vi "RT.vi"() -> ()   [LabVIEW 2015]
uses:
  _RT Global.vi
  Type/RT Loop Events.ctl
  Type/_RT Active Ch.ctl
  Type/_RT Mass Range.ctl
  Type/_RT Expt.ctl
  Type/_RT Parameter.ctl
  <vilib>/rvi/interface/nirviReadWriteControl/nirviReadWriteControl.xnode
  Type/_RW Status.ctl
  <vilib>/Utility/config.llb/NI_LVConfig.lvlib
  Type/_RT Res Type.ctl
  Type/_Run Mode.ctl
  <vilib>/Utility/config.llb/Write Key (Boolean).vi
  Type/_FPGA Indicator.ctl
  Type/_RT Serial Command.ctl
  <vilib>/NI_Real-Time Target Support.lvlib
  Type/_RT LED Num.ctl
  Type/_RT Instrument State.ctl
  Type/_LED States.ctl
  Type/_Pump Parameter.ctl
  Type/_LCD Line1 Msg.ctl
  Type/_LCD Line2 Msg.ctl
  Type/FPGA Typedef.ctl
  Type/_RT Command.ctl
  Type/TCP Packet Info.ctl
  Type/_RT Data.ctl
  FPGA Bitfiles/FPGA9607.lvbitx
  <vilib>/Utility/config.llb/Write Key (String).vi
  NiFpgaLv.dll
  <vilib>/Utility/error.llb/Error Cluster From Error Code.vi
  <vilib>/rvi/errors/niLvFpgaAdjustHostInterfaceError.vi
panel:
  in  "FW Version":string="1.7.0.170921.R"
  out "Speed":i32
  out "error":errorcluster
  out "LC Input Detected 3":bool
  out "LC Input Detected 2":bool
  in  "# Connections":u8
  out "RunMode":i32
  out "Running":bool
  out "Command":T1
  in  "Force Simulation (F)":bool
  out "Rt Loop Events":T2
  out "code":i32
  out "InstrState":T3=enum."Mass Spectrometer is Off"
  out "Fault":bool
  out "Ready":bool
  in  "RT Version":u32=2107170921
  out "FPGA Version":u32
  out "Time (s)":dbl
  out "Connected?":bool
  # "R&D"
  # "Run  Status"
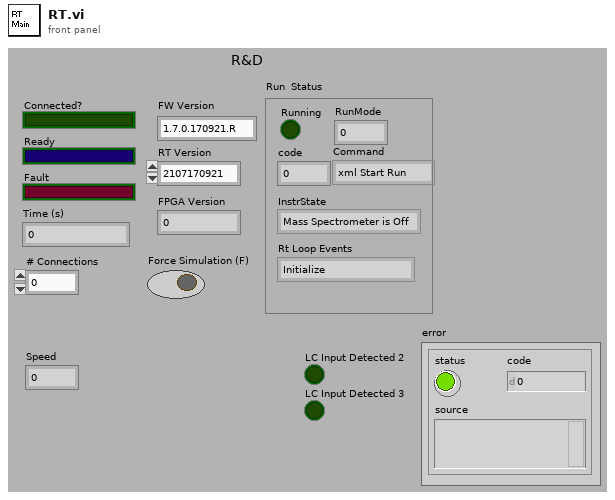
[diagram p1: front panel]
types:
  T1 = typedef "_RT Command.ctl" = enum16{"xml Start Run", "xml Start Actual Run", "xml Stop Run", "xml Runtime Update", "xml Get Status", "xml Get Table", "xml Set Table", "xml Get Configuration", "xml System Status", "xml Set LC Input Logic", "xml Get Data", "xml Get Info", "Start", "StartActualRun", "Stop", "Runtime Update", "Get Data", "Get Info", "Get Status", "Get Param", "Get Config", "Get Table", "Read ADC", "Set Oscillator", "Update Config", "Update Table", "Set All Pol", "Set Pol and DC", "Set Max Mass", "Toggle RP", "Toggle EL", "Set PIC", "Initialize Turbo", "Send Turbo Comm", "Close Turbo", "P1", "P2", "P3", "Send Serial", "Set LC Out", "Get LC In", "Read VAC", "Test Table", "Toggle Power", "Get Startup", "Set Startup", "Get ADC Table", "Set ADC Table", "Get Brief Status", "Get Detail Status", "Auxiliary Update", "Set CC Logics", "Set CC Input Logics", "Ignore Error", "invalid"}
  T2 = typedef "RT Loop Events.ctl" = enum16{"Initialize", "Wait for Connection", "Wait for Command", "Send Reply"}
  T3 = typedef "_RT Instrument State.ctl" = enum16{"Initializing", "Mass Spectrometer is Off", "Starting Up", "Turning Power Off", "Going to Standby", "Roughing Pump Ready", "Turning Turbo Off", "Turbo Startup", "Turbopump Ready", "Checking Vacuum", "Going to Ready", "Ready", "Running", "Source Standby", "Lost Communication", "Shutting Down", "Fault", "24V Standby", "Go to 24V Standby", "Turbopump Ready-Waiting"}
  T4 = typedef "_RT Parameter.ctl" = cluster{"RunMode":i32, "Initial Ch":T5[], "Sync":u8, "Expt":T6[], "EqTime(mS)":i32}
  T5 = typedef "_RT Active Ch.ctl" = cluster{"Start":i32, "Step":i32, "ChID":i32}
  T6 = typedef "_RT Expt.ctl" = cluster{"StartT(mS)":i32, "#Cycles":i32, "Scan Type":T7, "PauseT(uS)":i32, "Polarity":u8, "DelayT(mS)":i32, "Active Ch":T5[], "Mass Range":T8[]}
  T7 = typedef "_Run Mode.ctl" = enum16{"MRM (Q1/Q2)", "Q1 Scan", "Q1 SRM", "Q2 Scan", "Q2 SRM", "Product Scan", "Precursor Scan", "Neutral Loss", "Neutral Gain"}
  T8 = typedef "_RT Mass Range.ctl" = cluster{"Steps":i32, "Dwell(uS)":i32, "Resolution Type":T9, "Ramping Ch":T5[]}
  T9 = typedef "_RT Res Type.ctl" = u16
  T10 = cluster{"Rt Loop Events":T2, "Connection ID":refnum<k5>, "Parameter":T4, "Message Data":string, "Data Array":i32[], "Sequence Number":i32, "Command":T1, "error":errorcluster}
  T11 = typedef "FPGA Typedef.ctl" = refnum<k20>
  T12 = typedef "_RW Status.ctl" = enum8{"Done", "Do Read", "Do Write", "Set Latch1", "Set Latch2", "Set Latch3", "Set Latch4", "RP ON", "EL ON", "Serial Send", "Set LC Out", "Get LC In", "Read VAC", "Table Test", "Get Interlock", "Do Read2", "Do Write2"}
  T13 = typedef "_RT Serial Command.ctl" = cluster{"Port Type":u16, "baud rate (9600)":u32, "data bits (8)":u16, "stop bits (1)":u16, "parity (0:none)":u16, "DoRead":bool, "Command":string}
  T14 = typedef "_FPGA Indicator.ctl" = enum16{"Done", "Ready", "Count Available", "SendSerial", "LED State"}
  T15 = typedef "_Pump Parameter.ctl" = enum16{"Turn Pump Motor On", "Turn Pump Motor Off", "Read Pump Oil Deficiency", "Read Rotation Switch Point Attained", "Read Ele. Drive Over Temperature", "Read Pump Over Temperature", "Read Set Rotation Speed Attained", "Read Turbopump Accelerates", "Read Actual Rotation Speed in Hz", "Read Motor Current in A", "Read Operating Hours in h", "Read Motor Voltage in V", "Read Motor Power in W", "Set Rotation Speed Switchpoint in %", "Clear Error", "Read Error Code", "Read Bearing Temperature", "Read Hardware Version", "Read Firmware Version", "Read Operating Hours (Drive)", "Read Rotational Speed (rpm)", "Read Power Stage Temperature", "Read Electronics Temperature", "Read Upper Pump Temperature", "Read Motor Temperature", "Read Error Code History, 1", "Read Error Code History, 2", "Read Error Code History, 3", "Read Error Code History, 4", "Read Error Code History, 5", "Read Error Code History, 6", "Read Error Code History, 7", "Read Error Code History, 8", "Read Error Code History, 9", "Read Error Code History, 10"}
  T16 = typedef "TCP Packet Info.ctl" = cluster{"Packet Signature":string, "Sequence Number":i32, "Command":T1, "Data Message Size":u32, "Data Message Size":string, "Data Message":string, "Error Message Size":u32, "Error Message Size":string, "Error Message":string, "Checksum":u32, "Error Message":errorcluster, "Command ID":string}
  T17 = typedef "_RT Data.ctl" = cluster{"Info":string, "Data Array":i32[], "error out":errorcluster}
  T18 = typedef "_RT Startup Options.ctl" = cluster{"Door":bool, "Curtain":bool, "Pressure":bool, "Turbo":bool, "SysPoll":bool, "GasFlag":bool, "SourceExhaust":bool}
  T19 = typedef "_RT Instrument 2.ctl" = cluster{"Table":T20[], "Instrument":string[]}
  T20 = typedef "_RT Configuration 2.ctl" = cluster{"Name":string, "Ch#":u8, "Min":dbl, "Max":dbl, "Def+":dbl, "Def-":dbl, "Offset":dbl, "Slope":dbl, "Type":u8, "Description":string, "SettleT":dbl}
  T21 = typedef "NI_LVConfig.lvlib/Config Data RefNum.ctl" = refnum<k1>
  T22 = typedef "_RT LED Num.ctl" = enum8{"ReadKey", "ClearKeyBuffer", "ClearLCD", "BacklightOn"}
  T23 = typedef "_LED States.ctl" = enum8{"Idle", "Solid B", "Solid R", "Solid P", "Off B", "Off R", "Off P", "Off BRP", "Off RP", "Flash R&P", "Flash P"}
  T24 = typedef "_LCD Line2 Msg.ctl" = u16
  T25 = typedef "_LCD Line1 Msg.ctl" = u16
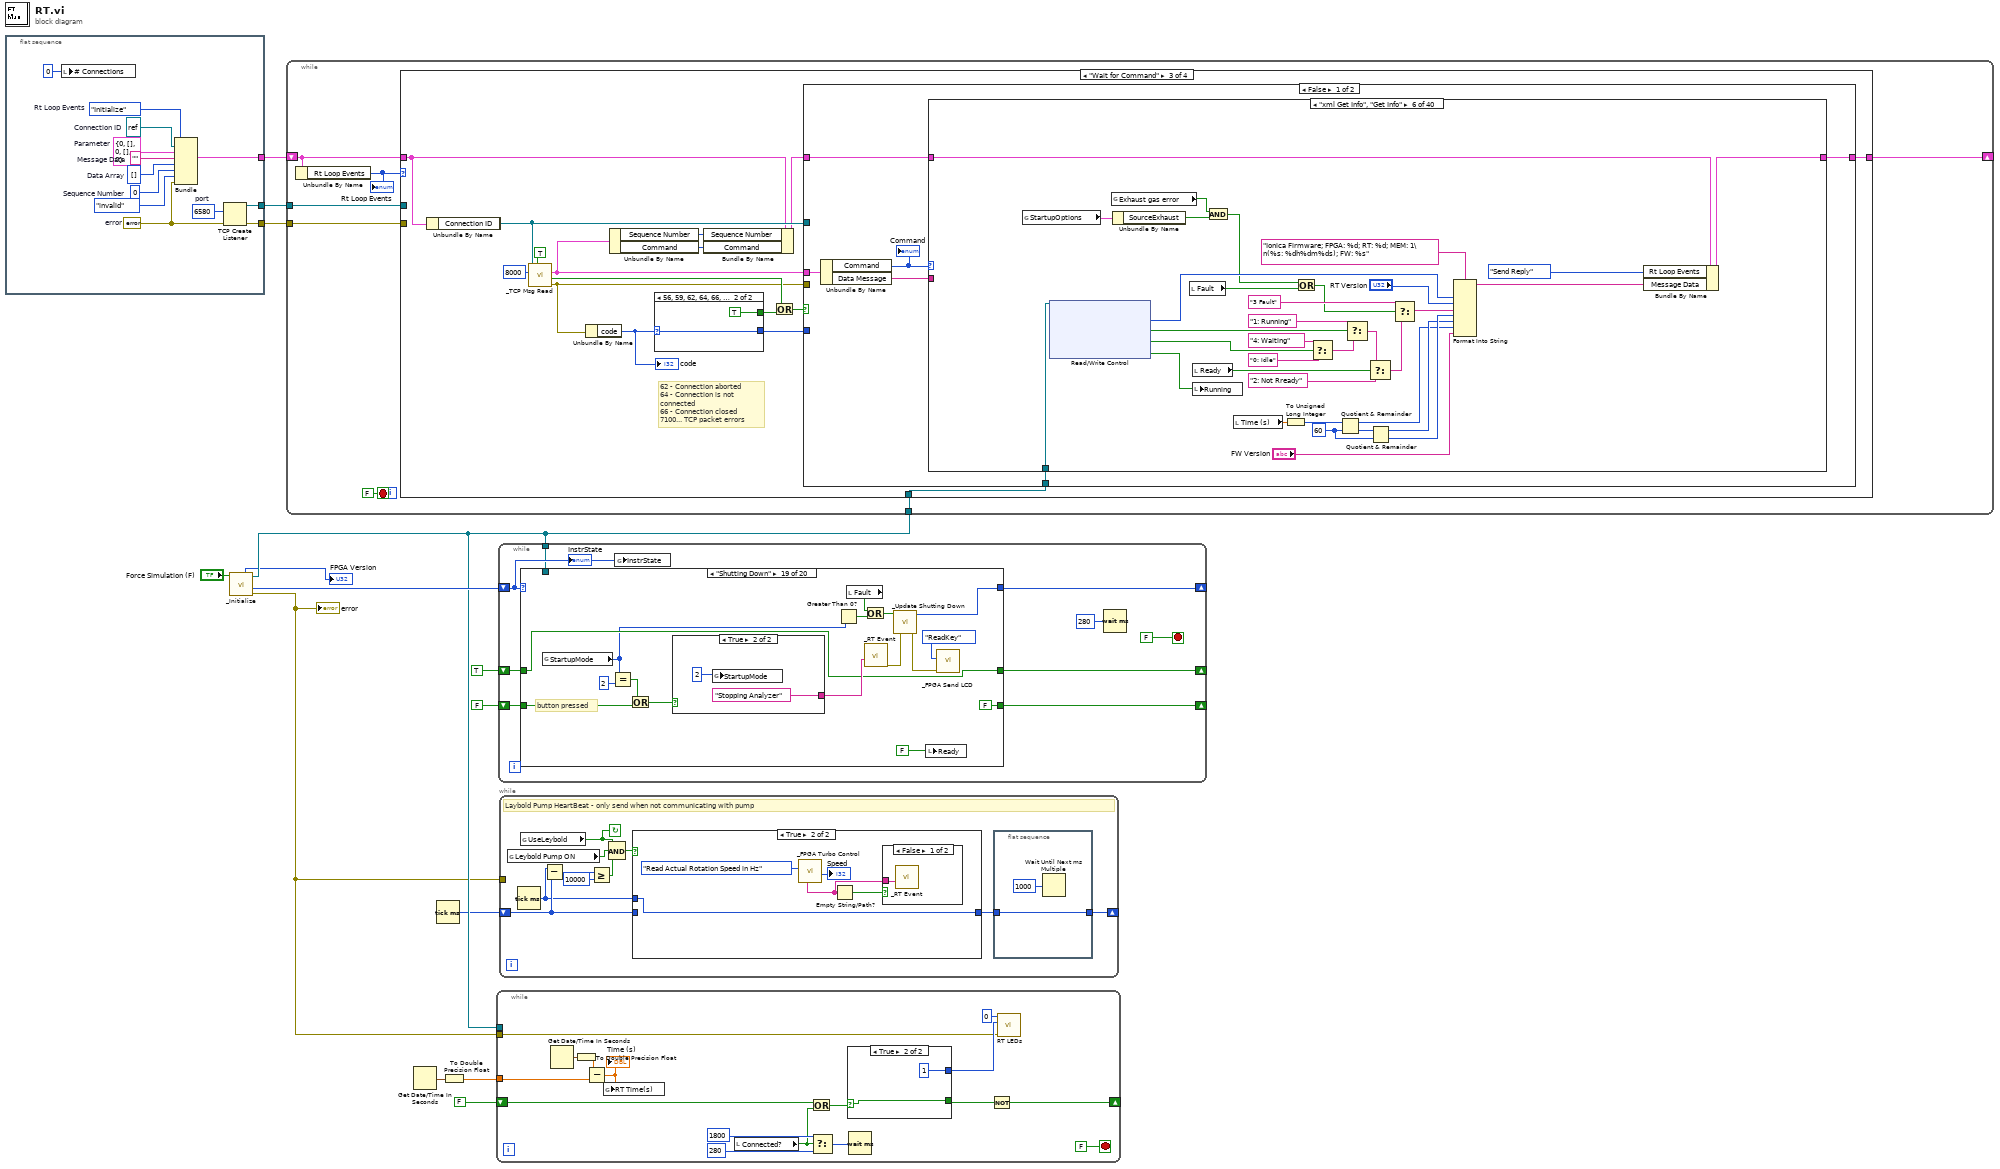
[diagram p0: block diagram]
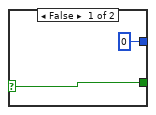
[diagram p4: hidden frame]
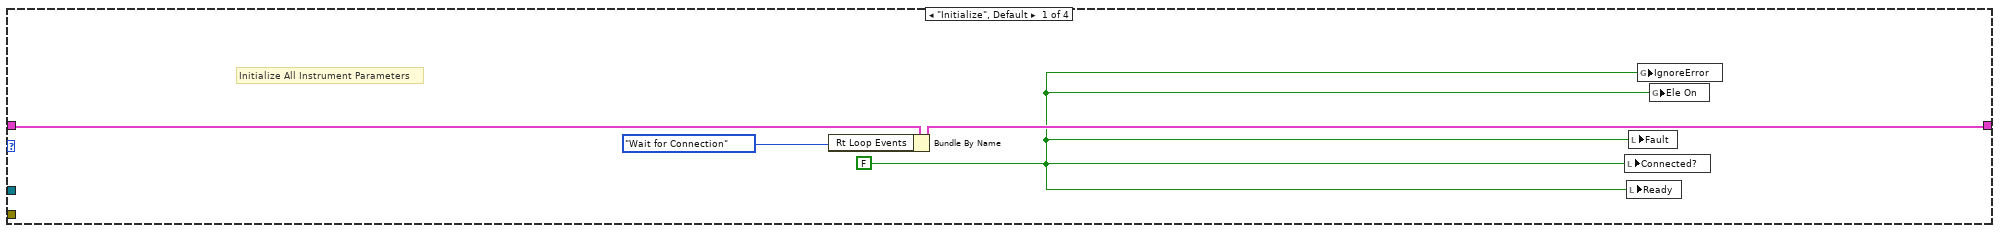
[diagram p5: hidden frame]
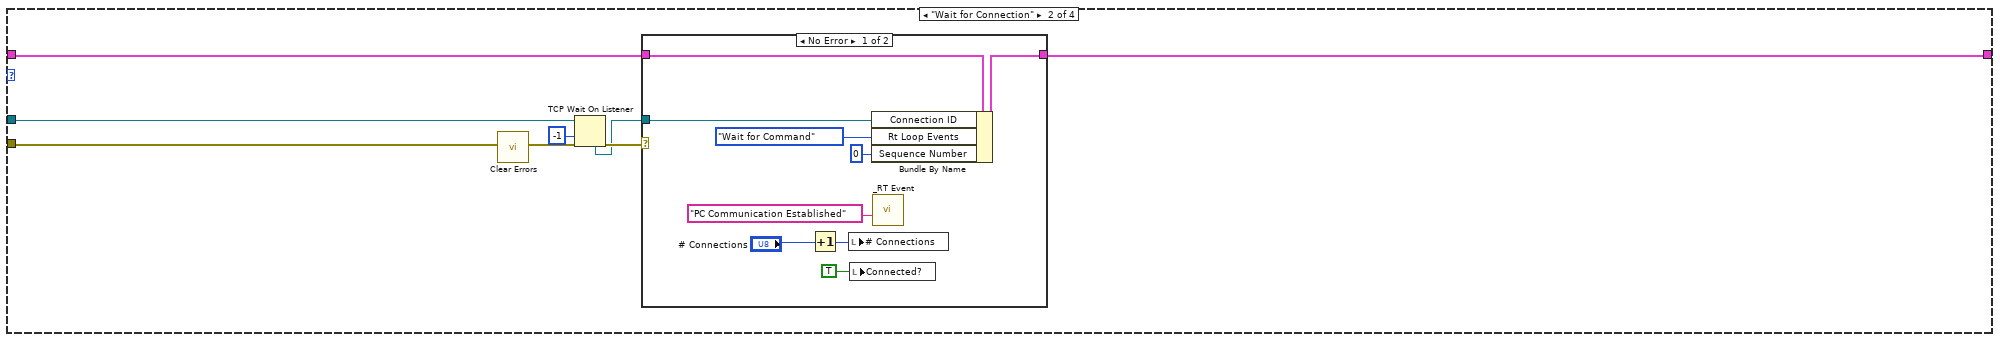
[diagram p6: hidden frame]
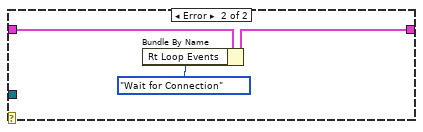
[diagram p7: hidden frame]
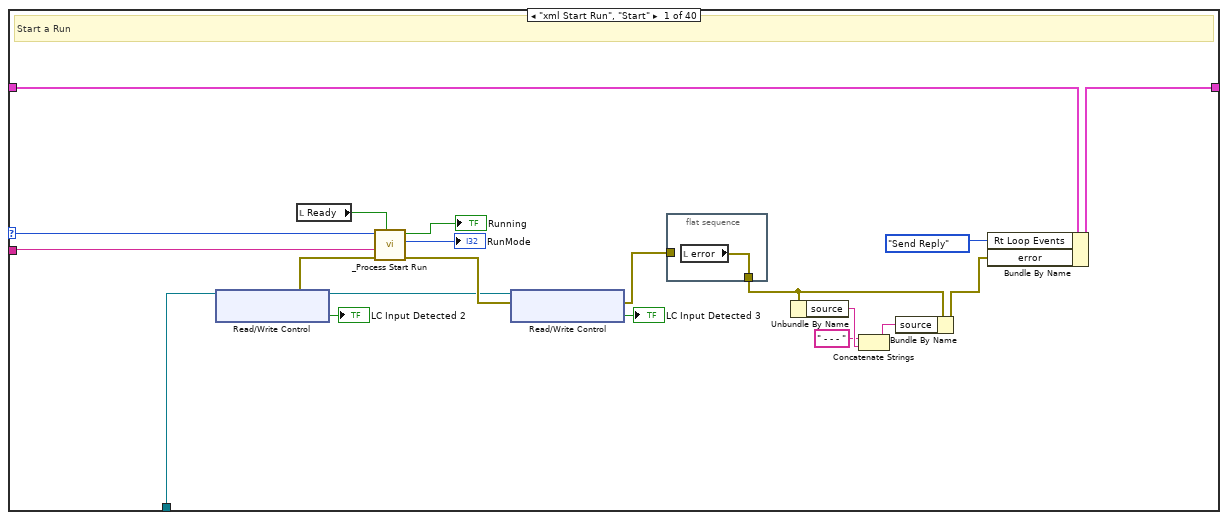
[diagram p8: hidden frame]
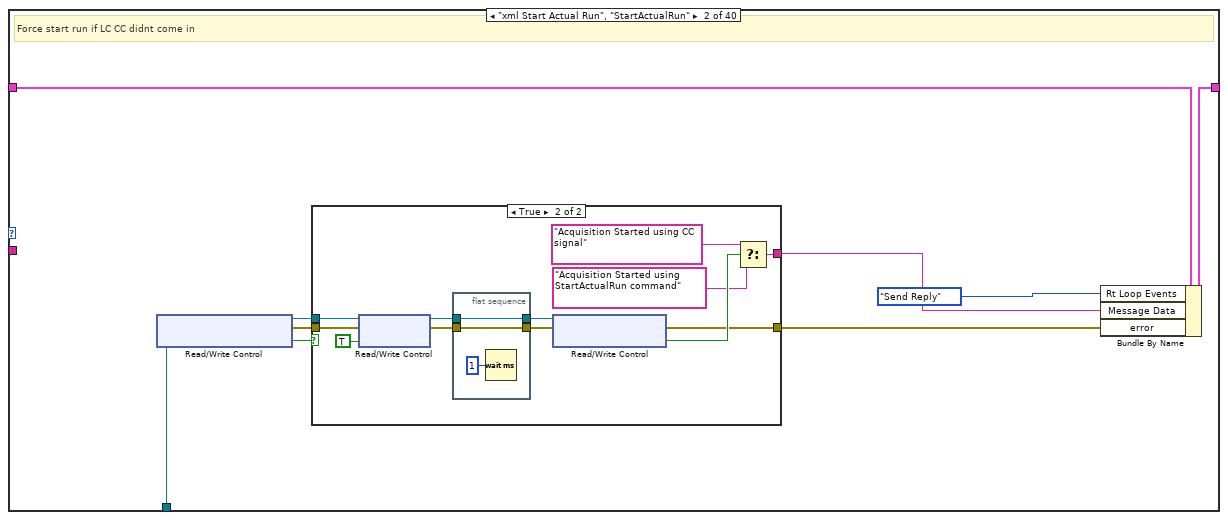
[diagram p9: hidden frame]
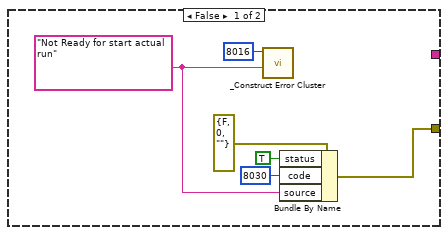
[diagram p10: hidden frame]
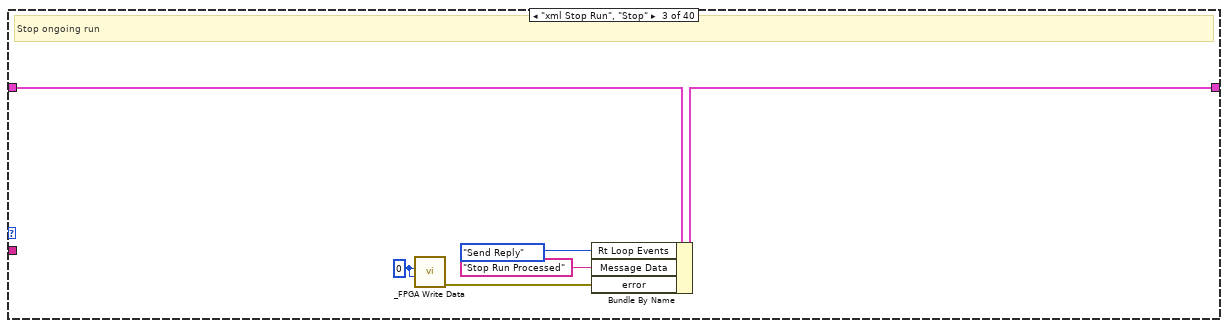
[diagram p11: hidden frame]
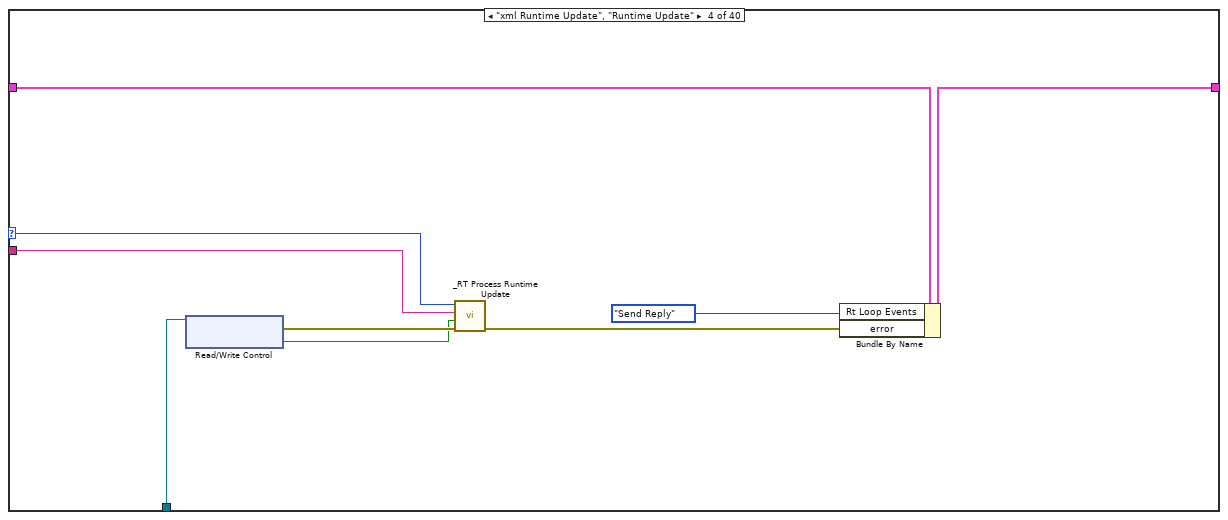
[diagram p12: hidden frame]
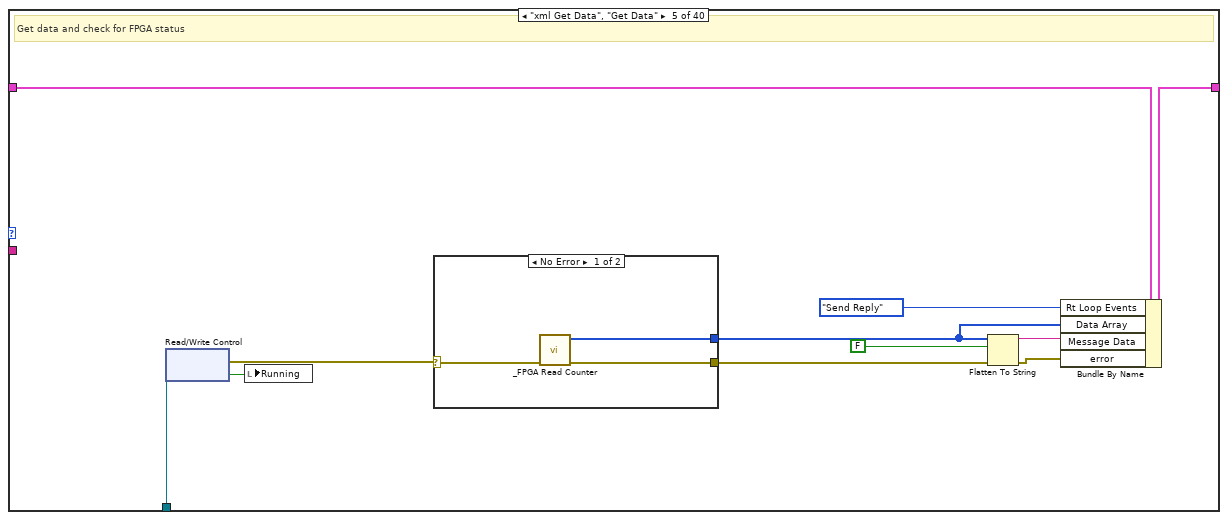
[diagram p13: hidden frame]
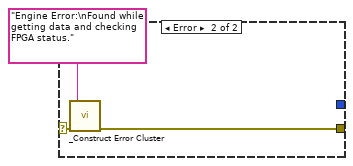
[diagram p14: hidden frame]
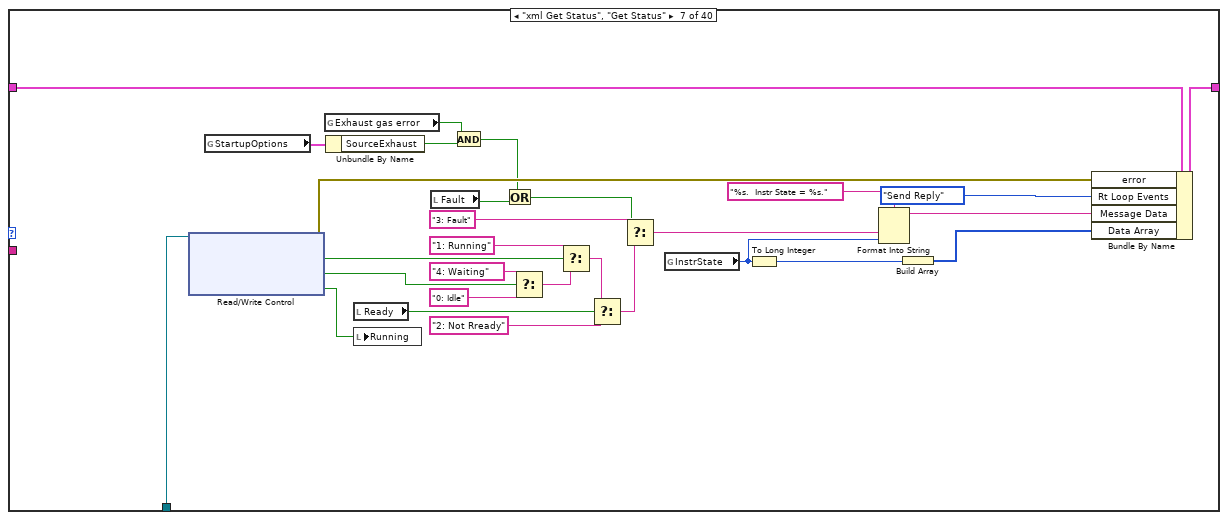
[diagram p15: hidden frame]
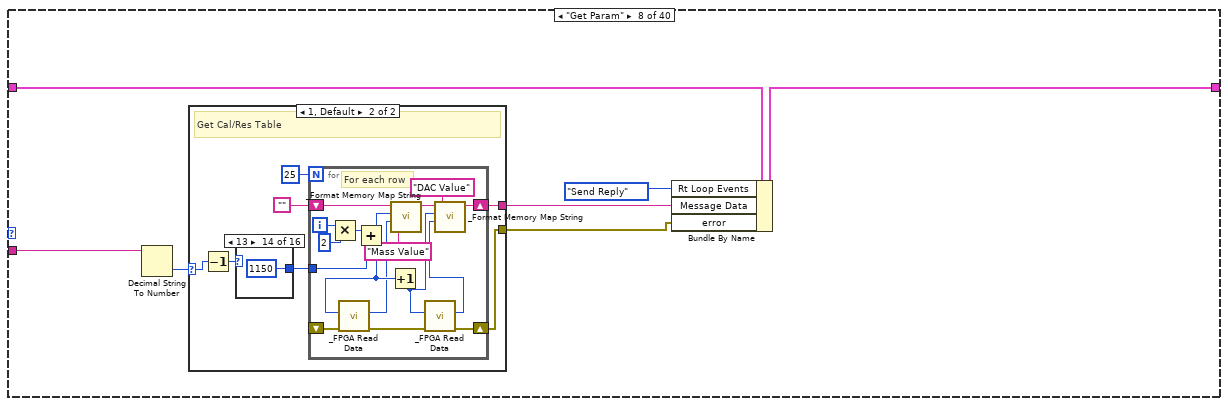
[diagram p16: hidden frame]
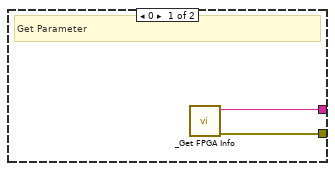
[diagram p17: hidden frame]
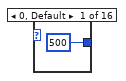
[diagram p18: hidden frame]
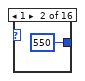
[diagram p19: hidden frame]
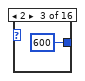
[diagram p20: hidden frame]
diagram:
  n1 = flat-sequence {
    tunnel: [w25] -> w14
    tunnel: [w21] -> w13
    tunnel: [w18] -> w5
    frame #0 {
      w19 = 0  # Sequence Number
      w20 = T4 {"RunMode"=0, "Initial Ch"=[], "Sync"=0, "Expt"=[], "EqTime(mS)"=0}  # Parameter
      w22 = u16 6580  # port
      w23 = i32[] []  # Data Array
      w24 = ""  # Message Data
      w15 = errorcluster {"status"=FALSE, "code"=0, "source"=""}  # error
      w26 = refnum<k5> refnum  # Connection ID
      w27 = RT_Loop_Events."Initialize"  # Rt Loop Events
      n2 = local write "# Connections"(u8 0 ("Disconnection#")) -> ()
      n3 = Bundle("Rt Loop Events"=w27, "Connection ID"=w26, "Parameter"=w20, "Message Data"=w24, "Data Array"=w23, "Sequence Number"=w19, "Command"=_RT_Command."invalid", "error"=w15) -> (w25:T10)  [unwired: 1 out]
      n4 = TCP Create Listener(8:w15, 10:w22) -> (0:w18:errorcluster, 3:w21:refnum<k5>)  [unwired: 4 out]
    }
  }
  n5 = call "_Initialize.vi"("Force Simulation (F)"="Force Simulation (F)") -> ("error"=w1:errorcluster, "InstrState"=w10:T3, "FPGA VI Reference Out"=w7:T11, "FPGA Version"=→"FPGA Version":u32)  [unwired: 7 in]
  "error" <- w1
  n6 = while {
    shift-right: [w28] -> _
    shift-left: w14 -> [w32]
    tunnel: w7 -> [w31]
    tunnel: w13 -> [w30]
    tunnel: w5 -> [w29]
    stop <- FALSE stop-if-true
    n7 = Unbundle By Name(w32) -> ("Rt Loop Events"=w33:T2)
    "Rt Loop Events" <- w33
    n8 = case shown="\"Wait for Command\"" w33 {
      tunnel: w32 -> [w37 w46 w59 w758]
      tunnel: [w36 w45 w73 w772] -> w28
      tunnel: w31 -> [_ _ w71 _]
      tunnel: w30 -> [_ w43 _ _]
      tunnel: w29 -> [_ w40 _ _]
      frame "Initialize", Default {
        w35 = FALSE ("Connected?")
        # "Initialize All Instrument Parameters"
        n9 = Bundle By Name(cluster=w37, "Rt Loop Events"=RT_Loop_Events."Wait for Connection") -> (w36:T10)
        n10 = local write "Connected?"(w35) -> ()
        n11 = local write "Ready"(w35) -> ()
        n12 = local write "Fault"(w35) -> ()
        n13 = global write "_RT Global.vi" "IgnoreError"(w35) -> ()
        n14 = global write "_RT Global.vi" "Ele On"(w35) -> ()
      }
      frame "Wait for Connection" {
        n15 = call <vilib>:"Clear Errors.vi"("error in (no error)"=w40) -> ("error out"=w39:errorcluster)  [unwired: 5 in, 1 out]
        n16 = TCP Wait On Listener(8:w39, 9:-1 ("timeout ms (wait forever: -1)"), 11:w43) -> (0:w44:errorcluster, 4:w42:refnum<k5>)  [unwired: 4 out]
        n17 = case shown="No Error" w44 {
          tunnel: w46 -> [w55 w58]
          tunnel: w42 -> [w53 _]
          tunnel: [w54 w56] -> w45
          frame No Error {
            n18 = Increment(x="# Connections") -> (x+1=w50:u8)
            n19 = local write "# Connections"(w50) -> ()
            n20 = local write "Connected?"(TRUE ("Connected?")) -> ()
            n21 = Bundle By Name(cluster=w55, "Connection ID"=w53, "Rt Loop Events"=RT_Loop_Events."Wait for Command", "Sequence Number"=0) -> (w54:T10)
            n22 = call "_RT Event.vi"("Event"="PC Communication Established") -> ()  [unwired: 2 in, 5 out]
          }
          frame Error {
            n23 = Bundle By Name(cluster=w58, "Rt Loop Events"=RT_Loop_Events."Wait for Connection") -> (w56:T10)
          }
        }
      }
      frame "Wait for Command" {
        # "62 - Connection aborted\n64 - Connection is not connected\n66 - Connection closed\n7100... TCP packet errors"
        n24 = Unbundle By Name(w59) -> ("Connection ID"=w69:refnum<k5>)
        n25 = call "_TCP Msg Read.vi"("RT"=TRUE, "timeout ms (10000)"=8000 ("millisecond multiple"), "connection ID"=w69) -> ("error out"=w60:errorcluster, "Read Timeout"=w66:bool, "Packet Info"=w62:T16)  [unwired: 1 in, 5 out]
        n26 = Unbundle By Name(w60) -> ("code"=w74:i32)
        "code" <- w74
        n27 = Unbundle By Name(w62) -> ("Sequence Number"=w64:i32, "Command"=w63:T1)
        n28 = case shown="56, 59, 62, 64, 66, 7100.., Default" w74 {
          selector: w74 -> [w753 w754]
          tunnel: [_ TRUE ("abort (F)")] -> w68
          tunnel: [w753 w754] -> w61
          frame 0 {
          }
          frame 56, 59, 62, 64, 66, 7100.., Default {
          }
        }
        n29 = Bundle By Name(cluster=w59, "Sequence Number"=w64, "Command"=w63) -> (w65:T10)
        n30 = Or(x=w66, y=w68) -> (x .or. y?=w70:bool)
        n31 = case shown="False" w70 {
          tunnel: w65 -> [w80 w733]
          tunnel: [w79 w732] -> w73
          tunnel: w62 -> [w77 _]
          tunnel: w71 -> [w78 _]
          tunnel: w69 -> [_ w731]
          tunnel: w61 -> [_ w730]
          tunnel: w60 -> [_ w729]
          frame False {
            n32 = Unbundle By Name(w77) -> ("Command"=w76:T1, "Data Message"=w75:string)
            "Command" <- w76
            n33 = case shown="\"xml Get Info\", \"Get Info\"" w76 {
              selector: w76 -> [w97 _ _ w140 _ _ _ _ w276 _ _ _ w337 w382 _ _ _ _ _ _ _ _ _ _ _ _ _ _ _ _ _ _ _ _ _ _ w694 _ _ w722]
              tunnel: w75 -> [w96 _ _ w141 _ _ _ w231 _ _ w300 w327 w340 w381 w404 w425 w429 w440 w455 w471 w479 w487 w499 w509 _ _ w546 w574 _ w587 _ w615 w622 _ w678 w689 w699 w712 w721 _]
              tunnel: w80 -> [w99 w109 w137 w145 w157 w198 w227 w234 w282 w294 w306 w324 w343 w386 w401 w422 w433 w442 w453 w468 w476 w484 w497 w513 w522 w529 w556 w577 w583 w597 w603 w612 w639 w672 w683 w692 w701 w715 w718 w725]
              tunnel: [w98 w108 w136 w144 w156 w197 w226 w233 w281 w293 w305 w323 w342 w384 w400 w421 w432 w441 w452 w467 w475 w483 w496 w512 w521 w528 w555 w576 w582 w596 w602 w611 w638 w671 w682 w691 w700 w714 w717 w724] -> w79
              tunnel: w78 -> [w92 w107 _ w143 w153 w195 w224 _ _ _ w304 _ _ _ _ _ _ _ w451 _ _ _ w495 _ _ _ w531 _ _ _ _ _ _ w656 _ _ _ _ _ _]
              frame "xml Start Run", "Start" {
                # "Start a Run"
                n34 = xnode "Read/Write Control"("FPGA VI Reference In"=w92) -> ("FPGA VI Reference Out"=w89:T11, "error out"=w91:errorcluster, "LC Input Detected"=→"LC Input Detected 2":bool)  [unwired: 1 in]
                n35 = local read "Ready"() -> (w95:bool)
                n36 = call "_Process Start Run.vi"("Ready"=w95, "Error In"=w91, "binary string"=w96, "Command"=w97) -> ("Error Out"=w90:errorcluster, "RunMode"=→"RunMode":i32, "Running"=→"Running":bool)  [unwired: 5 in]
                n37 = xnode "Read/Write Control"("FPGA VI Reference In"=w89, "error in"=w90) -> ("error out"=w85:errorcluster, "LC Input Detected"=→"LC Input Detected 3":bool)  [unwired: 1 out]
                n38 = flat-sequence {
                  tunnel: [w101] -> w84
                  tunnel: w85 -> [_]
                  frame #0 {
                    n39 = local read "error"() -> (w101:errorcluster)
                  }
                }
                n40 = Unbundle By Name(w84) -> ("source"=w83:string)
                n41 = Concatenate Strings(" - - - " ("string"), w83) -> (w82:string)
                n42 = Bundle By Name(cluster=w84, "source"=w82) -> (w86:errorcluster)
                n43 = Bundle By Name(cluster=w99, "Rt Loop Events"=RT_Loop_Events."Send Reply", "error"=w86) -> (w98:T10)
              }
              frame "xml Start Actual Run", "StartActualRun" {
                # "Force start run if LC CC didnt come in"
                n44 = xnode "Read/Write Control"("FPGA VI Reference In"=w107) -> ("FPGA VI Reference Out"=w104:T11, "error out"=w105:errorcluster, "Ready to Acquire Data"=w106:bool)  [unwired: 1 in]
                n45 = case shown="True" w106 {
                  tunnel: w105 -> [_ w126]
                  tunnel: w104 -> [_ w128]
                  tunnel: [w111 w118] -> w103
                  tunnel: [_ w117] -> w102
                  frame False {
                    w112 = "Not Ready for start actual run"
                    n46 = call "_Construct Error Cluster.vi"("reason"=w112, "errorCode"=8016) -> ()  [unwired: 2 in, 4 out]
                    n47 = Bundle By Name(cluster=errorcluster {"status"=FALSE, "code"=0, "source"=""} ("error constant"), "status"=TRUE, "code"=8030, "source"=w112) -> (w111:errorcluster)
                  }
                  frame True {
                    n48 = xnode "Read/Write Control"("FPGA VI Reference In"=w128, "error in"=w126, "ForceStart"=TRUE ("Start")) -> ("FPGA VI Reference Out"=w119:T11, "error out"=w121:errorcluster)
                    n49 = flat-sequence {
                      tunnel: [w131] -> w122
                      tunnel: w121 -> [w131]
                      tunnel: [w130] -> w120
                      tunnel: w119 -> [w130]
                      frame #0 {
                        n50 = Wait (ms)(milliseconds to wait=u32 1) -> ()  [unwired: 1 out]
                      }
                    }
                    n51 = xnode "Read/Write Control"("FPGA VI Reference In"=w120, "error in"=w122) -> ("error out"=w118:errorcluster, "LC Input Detected"=w125:bool)  [unwired: 1 out]
                    n52 = Select(t="Acquisition Started using CC signal" ("source"), s=w125, f="Acquisition Started using StartActualRun command" ("source")) -> (s? t:f=w117:string)
                  }
                }
                n53 = Bundle By Name(cluster=w109, "Rt Loop Events"=RT_Loop_Events."Send Reply", "Message Data"=w102, "error"=w103) -> (w108:T10)
              }
              frame "xml Stop Run", "Stop" {
                w134 = u16 0 ("Address")
                # "Stop ongoing run"
                n54 = call "_FPGA Write Data.vi"("Data"=w134, "Address"=w134) -> ("error out"=w133:errorcluster)  [unwired: 4 in, 2 out]
                n55 = Bundle By Name(cluster=w137, "Rt Loop Events"=RT_Loop_Events."Send Reply", "Message Data"="Stop Run Processed" ("string"), "error"=w133) -> (w136:T10)
              }
              frame "xml Runtime Update", "Runtime Update" {
                n56 = xnode "Read/Write Control"("FPGA VI Reference In"=w143) -> ("error out"=w142:errorcluster, "Acquiring Data"=w138:bool)  [unwired: 1 in, 1 out]
                n57 = call "_RT Process Runtime Update.vi"("Error In"=w142, "Acquiring Data"=w138, "binary string"=w141, "Command"=w140) -> ("Error Out"=w139:errorcluster)  [unwired: 7 in]
                n58 = Bundle By Name(cluster=w145, "Rt Loop Events"=RT_Loop_Events."Send Reply", "error"=w139) -> (w144:T10)
              }
              frame "xml Get Data", "Get Data" {
                # "Get data and check for FPGA status"
                n59 = xnode "Read/Write Control"("FPGA VI Reference In"=w153) -> ("error out"=w154:errorcluster, "Running"=w155:bool)  [unwired: 1 in, 1 out]
                n60 = local write "Running"(w155) -> ()
                n61 = case shown="No Error" w154 {
                  selector: w154 -> [w160 w163]
                  tunnel: [w158 _] -> w147
                  tunnel: [w159 w161] -> w150
                  frame No Error {
                    n62 = call "_FPGA Read Counter.vi"("error in (no error)"=w160) -> ("error out"=w159:errorcluster, "Data"=w158:u32[])  [unwired: 8 in, 1 out]
                  }
                  frame Error {
                    n63 = call "_Construct Error Cluster.vi"("error in"=w163, "reason"="Engine Error:\nFound while getting data and checking FPGA status.") -> ("error out"=w161:errorcluster)  [unwired: 2 in, 3 out]
                  }
                }
                n64 = Flatten To String(anything=w147, prepend array or string size? (T)=FALSE, error in (no error)=w150) -> (data string=w152:string, error out=w149:errorcluster)  [unwired: 1 in, 1 out]
                n65 = Bundle By Name(cluster=w157, "Rt Loop Events"=RT_Loop_Events."Send Reply", "Data Array"=w147, "Message Data"=w152, "error"=w149) -> (w156:T10)
              }
              frame "xml Get Info", "Get Info" {
                w190 = u32 60 ("y")
                n66 = global read "_RT Global.vi" "StartupOptions"() -> (w168:T18)
                n67 = xnode "Read/Write Control"("FPGA VI Reference In"=w195) -> ("Version"=w194:u32, "Acquiring Data"=w174:bool, "Ready to Acquire Data"=w173:bool, "Running"=w172:bool)  [unwired: 1 in, 2 out]
                n68 = global read "_RT Global.vi" "Exhaust gas error"() -> (w166:bool)
                n69 = Unbundle By Name(w168) -> ("SourceExhaust"=w167:bool)
                n70 = local read "Fault"() -> (w170:bool)
                n71 = local read "Ready"() -> (w175:bool)
                n72 = local write "Running"(w172) -> ()
                n73 = And(x=w166, y=w167) -> (x .and. y?=w165:bool)
                n74 = local read "Time (s)"() -> (w186:dbl)
                n75 = To Unsigned Long Integer(number=w186) -> (unsigned 32bit integer=w188:u32)
                n76 = Or(x=w165, y=w170) -> (x .or. y?=w169:bool)
                n77 = Select(t="4: Waiting", s=w173, f="0: Idle") -> (s? t:f=w181:string)
                n78 = Quotient & Remainder(x=w188, y=w190) -> (x-y*floor(x/y)=w191:u32, floor(x/y)=w189:u32)
                n79 = Select(t="1: Running", s=w174, f=w181) -> (s? t:f=w183:string)
                n80 = Select(t=w183, s=w175, f="2: Not Rready") -> (s? t:f=w178:string)
                n81 = Quotient & Remainder(x=w189, y=w190) -> (x-y*floor(x/y)=w192:u32, floor(x/y)=w193:u32)
                n82 = Select(t="3 Fault", s=w169, f=w178) -> (s? t:f=w171:string)
                n83 = Format Into String(format string="Ionica Firmware; FPGA: %d; RT: %d; MEM: 1\n(%s: %dh%dm%ds); FW: %s", w194, "RT Version", w171, w193, w192, w191, "FW Version") -> (resulting string=w184:string)  [unwired: 2 in, 1 out]
                n84 = Bundle By Name(cluster=w198, "Rt Loop Events"=RT_Loop_Events."Send Reply", "Message Data"=w184) -> (w197:T10)
              }
              frame "xml Get Status", "Get Status" {
                n85 = xnode "Read/Write Control"("FPGA VI Reference In"=w224) -> ("error out"=w206:errorcluster, "Acquiring Data"=w208:bool, "Ready to Acquire Data"=w205:bool, "Running"=w207:bool)  [unwired: 1 in, 1 out]
                n86 = global read "_RT Global.vi" "StartupOptions"() -> (w202:T18)
                n87 = global read "_RT Global.vi" "Exhaust gas error"() -> (w200:bool)
                n88 = Unbundle By Name(w202) -> ("SourceExhaust"=w201:bool)
                n89 = local read "Ready"() -> (w209:bool)
                n90 = local write "Running"(w207) -> ()
                n91 = local read "Fault"() -> (w203:bool)
                n92 = And(x=w200, y=w201) -> (x .and. y?=w199:bool)
                n93 = Or(x=w199, y=w203) -> (x .or. y?=w204:bool)
                n94 = Select(t="4: Waiting", s=w205, f="0: Idle") -> (s? t:f=w216:string)
                n95 = Select(t="1: Running", s=w208, f=w216) -> (s? t:f=w218:string)
                n96 = Select(t=w218, s=w209, f="2: Not Rready") -> (s? t:f=w213:string)
                n97 = Select(t="3: Fault", s=w204, f=w213) -> (s? t:f=w210:string)
                n98 = global read "_RT Global.vi" "InstrState"() -> (w221:T3)
                n99 = To Long Integer(number=w221) -> (32bit integer=w223:i32)
                n100 = Format Into String(format string="%s.  Instr State = %s.", w210, w221) -> (resulting string=w219:string)  [unwired: 2 in, 1 out]
                n101 = Build Array(w223) -> (w222:i32[])
                n102 = Bundle By Name(cluster=w227, "error"=w206, "Rt Loop Events"=RT_Loop_Events."Send Reply", "Message Data"=w219, "Data Array"=w222) -> (w226:T10)
              }
              frame "Get Param" {
                n103 = Decimal String To Number(string=w231) -> (number=w230:i32)  [unwired: 3 out]
                n104 = case shown="1, Default" w230 {
                  selector: w230 -> [_ w243]
                  tunnel: [w236 w239] -> w229
                  tunnel: [w235 w237] -> w228
                  frame 0 {
                    # "Get Parameter"
                    n105 = call "_Get FPGA Info.vi"() -> ("error out"=w235:errorcluster, "Info"=w236:string)  [unwired: 2 in, 4 out]
                  }
                  frame 1, Default {
                    # "Get Cal/Res Table"
                    n106 = Decrement(x=w243) -> (x-1=w242:i32)
                    n107 = case shown="13" w242 {
                      tunnel: [u16 500 ("Addr Offset") u16 550 ("Addr Offset") u16 600 ("Addr Offset") u16 650 ("Addr Offset") u16 700 ("Addr Offset") u16 750 ("Addr Offset") u16 800 ("Addr Offset") u16 850 ("Addr Offset") u16 900 ("Addr Offset") u16 950 ("Addr Offset") u16 1000 ("Addr Offset") u16 1050 ("Addr Offset") u16 1100 ("Addr Offset") u16 1150 ("Addr Offset") u16 1200 ("Addr Offset") u16 1250 ("Addr Offset")] -> w240
                      frame 0, Default {
                      }
                      frame 1 {
                      }
                      frame 2 {
                      }
                      frame 3 {
                      }
                      frame 4 {
                      }
                      frame 5 {
                      }
                      frame 6 {
                      }
                      frame 7 {
                      }
                      frame 8 {
                      }
                      frame 9 {
                      }
                      frame 10 {
                      }
                      frame 11 {
                      }
                      frame 12 {
                      }
                      frame 13 {
                      }
                      frame 14 {
                      }
                      frame 15 {
                      }
                    }
                    n108 = for {
                      N: 25 -> [_]
                      shift-right: [w249] -> w239
                      shift-left: "" -> [w252]
                      tunnel: w240 -> [w256]
                      shift-right: [w253] -> w237
                      shift-left: _ -> [w254]
                      i -> [w259]
                      # "For each row"
                      n109 = Multiply(x=w259, y=2) -> (x*y=w257:i32)
                      n110 = Add(x=w257, y=w256) -> (x+y=w251:i32)
                      n111 = call "_FPGA Read Data.vi"("error in"=w254, "Address"=w251) -> ("error out"=w255:errorcluster, "Data"=w250:u32)  [unwired: 3 in, 1 out]
                      n112 = Increment(x=w251) -> (x+1=w247:i32)
                      n113 = call "_Format Memory Map String.vi"("User value"="Mass Value", "Data"=w250, "Address"=w251, "String In"=w252) -> ("String Out"=w248:string)  [unwired: 3 out]
                      n114 = call "_FPGA Read Data.vi"("error in"=w255, "Address"=w247) -> ("error out"=w253:errorcluster, "Data"=w246:u32)  [unwired: 3 in, 1 out]
                      n115 = call "_Format Memory Map String.vi"("User value"="DAC Value", "Data"=w246, "Address"=w247, "String In"=w248) -> ("String Out"=w249:string)  [unwired: 3 out]
                    }
                  }
                }
                n116 = Bundle By Name(cluster=w234, "Rt Loop Events"=RT_Loop_Events."Send Reply", "Message Data"=w229, "error"=w228) -> (w233:T10)
              }
              frame "xml Get Configuration", "Get Config" {
                n117 = global read "_RT Global.vi" "Configuration 2"() -> (w279:T19)
                n118 = case shown="\"xml Get Configuration\", Default" w276 {
                  tunnel: w279 -> [w283 w288]
                  tunnel: [w284 w287] -> w278
                  tunnel: [w285 w286] -> w277
                  frame "xml Get Configuration", Default {
                    n119 = call "_Write XML Configuration.vi"("Configuration"=w283) -> ("error out"=w285:errorcluster, "XML String"=w284:string)  [unwired: 1 in, 4 out]
                  }
                  frame "Get Config" {
                    n120 = Flatten To String(anything=w288) -> (data string=w287:string, error out=w286:errorcluster)  [unwired: 1 in, 3 out]
                  }
                }
                n121 = Bundle By Name(cluster=w282, "Rt Loop Events"=RT_Loop_Events."Send Reply", "Message Data"=w278, "error"=w277) -> (w281:T10)
              }
              frame "Read ADC" {
                # "Read ADC"
                n122 = call "_FPGA Read ADC.vi"() -> ("error out"=w289:errorcluster, "Running"=w291:bool, "ADC Values"=w290:i32[])  [unwired: 3 in, 4 out]
                n123 = local write "Running"(w291) -> ()
                n124 = Bundle By Name(cluster=w294, "Rt Loop Events"=RT_Loop_Events."Send Reply", "Data Array"=w290, "error"=w289) -> (w293:T10)
              }
              frame "Set Oscillator" {
                # "Set Oscillator"
                n125 = Unflatten From String(type=u32[] [], binary string=w300) -> (value=w302:u32[])  [unwired: 1 in, 4 out]
                n126 = xnode "Read/Write Control"("FPGA VI Reference In"=w304) -> ("error out"=w303:errorcluster, "Running"=w299:bool)  [unwired: 1 in, 1 out]
                n127 = local write "Running"(w299) -> ()
                n128 = Index Array(array=w302) -> (element #1=w298:u32, element #2=w297:u32, element #3=w296:u32)  [unwired: 3 in]
                n129 = call "_FPGA Set Oscillator.vi"("Param 3"=w296, "error in"=w303, "Param 2"=w297, "Param 1"=w298) -> ("error out"=w295:errorcluster)  [unwired: 1 in, 3 out]
                n130 = Bundle By Name(cluster=w306, "Rt Loop Events"=RT_Loop_Events."Send Reply", "error"=w295) -> (w305:T10)
              }
              frame "Update Config" {
                # "Max mass should be the same for channels 1, 2, 4,5 so we will just take the first one"
                # "Set Configuration"
                n131 = global read "_RT Global.vi" "Configuration 2"() -> (w326:T19)
                n132 = Unflatten From String(type=w326, binary string=w327) -> (value=w309:T19, error out=w320:errorcluster)  [unwired: 1 in, 3 out]
                n133 = Unbundle By Name(w309) -> ("Instrument"=w319:string[])
                n134 = Unbundle By Name(w309) -> ("Table"=w308:T20[])
                n135 = for {
                  tunnel: w308 -> [w331] mode=indexing
                  stop <- w328 stop-if-true
                  n136 = Unbundle By Name(w331) -> ("Ch#"=w329:u8, "Max"=w330:dbl)
                  n137 = case shown="0, Default" w329 {
                    tunnel: w330 -> [_ w334]
                    tunnel: [FALSE ("x >= 0?") TRUE ("x >= 0?")] -> w328
                    frame 0, Default {
                    }
                    frame 1 {
                      n138 = global write "_RT Global.vi" "Max Mass"(w334) -> ()
                    }
                  }
                }
                n139 = Index Array(array=w319, index=2) -> (element=w314:string)
                n140 = call "_Convert Model Name.vi"("Model"=w314) -> ("SingleSource"=w313:bool)  [unwired: 1 in, 1 out]
                n141 = Match Pattern(string=w314, regular expression="Simulation") -> (offset past match=w317:i32)  [unwired: 4 out]
                n142 = call "_Get Startup File.vi"("FileName"="Config" ("key")) -> ("FilePath"=w312:path)
                n143 = Greater Or Equal To 0?(x=w317) -> (x >= 0?=w315:bool)
                n144 = global write "_RT Global.vi" "Configuration 2"(w309) -> ()
                n145 = global write "_RT Global.vi" "Single Source"(w313) -> ()
                n146 = Write to Binary File(file (use dialog)=w312, data=w309, error in=w320) -> (refnum out=w321:refnum<file>, error out=w322:errorcluster)  [unwired: 4 out]
                n147 = global write "_RT Global.vi" "Simulation"(w315) -> ()
                n148 = Close File(refnum=w321, error in=w322) -> (error out=w310:errorcluster)  [unwired: 1 out]
                n149 = Bundle By Name(cluster=w324, "Rt Loop Events"=RT_Loop_Events."Send Reply", "error"=w310) -> (w323:T10)
              }
              frame "xml Get Table", "Get Table" {
                # "Get a Calibration/Resolution Table"
                n150 = Decimal String To Number(string=w340) -> (number=w335:i32)  [unwired: 3 out]
                n151 = case shown="0, Default" w335 {
                  selector: w335 -> [w349 w351 w353 w355 w357 w359 w361 w363 w365 w367 w369 w371 w373 w375 w377 w379]
                  tunnel: [w350 w352 w354 w356 w358 w360 w362 w364 w366 w368 w370 w372 w374 w376 w378 w380] -> w339
                  tunnel: [w349 w351 w353 w355 w357 w359 w361 w363 w365 w367 w369 w371 w373 w375 w377 w379] -> w336
                  frame 0, Default {
                    n152 = global read "_RT Global.vi" "Q1 Cal"() -> (w350:dbl[][])
                  }
                  frame 1 {
                    n153 = global read "_RT Global.vi" "Q2 Cal"() -> (w352:dbl[][])
                  }
                  frame 2 {
                    n154 = global read "_RT Global.vi" "Q1 -Cal"() -> (w354:dbl[][])
                  }
                  frame 3 {
                    n155 = global read "_RT Global.vi" "Q2 -Cal"() -> (w356:dbl[][])
                  }
                  frame 4 {
                    n156 = global read "_RT Global.vi" "Q1 Res Hi"() -> (w358:dbl[][])
                  }
                  frame 5 {
                    n157 = global read "_RT Global.vi" "Q2 Res Hi"() -> (w360:dbl[][])
                  }
                  frame 6 {
                    n158 = global read "_RT Global.vi" "Q1 Res Med"() -> (w362:dbl[][])
                  }
                  frame 7 {
                    n159 = global read "_RT Global.vi" "Q2 Res Med"() -> (w364:dbl[][])
                  }
                  frame 8 {
                    n160 = global read "_RT Global.vi" "Q1 Res Lo"() -> (w366:dbl[][])
                  }
                  frame 9 {
                    n161 = global read "_RT Global.vi" "Q2 Res Lo"() -> (w368:dbl[][])
                  }
                  frame 10 {
                    n162 = global read "_RT Global.vi" "Q1 -Res Hi"() -> (w370:dbl[][])
                  }
                  frame 11 {
                    n163 = global read "_RT Global.vi" "Q2 -Res Hi"() -> (w372:dbl[][])
                  }
                  frame 12 {
                    n164 = global read "_RT Global.vi" "Q1 -Res Med"() -> (w374:dbl[][])
                  }
                  frame 13 {
                    n165 = global read "_RT Global.vi" "Q2 -Res Med"() -> (w376:dbl[][])
                  }
                  frame 14 {
                    n166 = global read "_RT Global.vi" "Q1 -Res Lo"() -> (w378:dbl[][])
                  }
                  frame 15 {
                    n167 = global read "_RT Global.vi" "Q2 -Res Lo"() -> (w380:dbl[][])
                  }
                }
                n168 = case shown="\"xml Get Table\", Default" w337 {
                  tunnel: w339 -> [w346 w348]
                  tunnel: [w345 w347] -> w338
                  tunnel: w336 -> [w344 _]
                  frame "xml Get Table", Default {
                    n169 = call "_Write XML Table.vi"("Table Type"=w344, "Table (2D-DBL)"=w346) -> ("XML String"=w345:string)  [unwired: 1 in, 4 out]
                  }
                  frame "Get Table" {
                    n170 = Flatten To String(anything=w348) -> (data string=w347:string)  [unwired: 1 in, 4 out]
                  }
                }
                n171 = Bundle By Name(cluster=w343, "Rt Loop Events"=RT_Loop_Events."Send Reply", "Message Data"=w338) -> (w342:T10)
              }
              frame "xml Set Table", "Update Table" {
                # "Update a Calibration/Resolution Table"
                n172 = call "_RT Process Set Table.vi"("Data"=w381, "Command"=w382) -> ("Error Out"=w383:errorcluster)  [unwired: 9 in]
                n173 = Bundle By Name(cluster=w386, "Rt Loop Events"=RT_Loop_Events."Send Reply", "error"=w383) -> (w384:T10)
              }
              frame "Set All Pol" {
                # "Set Source Polarity:"
                # "Set CEM POL for Latch4"
                # "Set S1 POL, S2 POL for Latch3"
                # "Set COR POL, CUR POL for Latch2"
                n174 = Type Cast(type=u16 0, x=w404) -> (*(type *) &x=w390:u16)
                n175 = Greater Than 0?(x=w390) -> (x > 0?=w389:bool)
                n176 = Number To Boolean Array(number=u16 0) -> (Boolean array=w394:bool[])
                n177 = Replace Array Subset(array=w394, new element #1=w389, index #1=0 ("index"), new element #2=w389, index #2=1 ("index")) -> (w391:bool[])
                n178 = Boolean Array To Number(Boolean array=w391) -> (number=w388:u16)
                n179 = call "_FPGA Set Digi Line.vi"("States"=w388, "Line (Set Latch1)"=_RW_Status."Set Latch2" ("Write Mode (Do Write)")) -> ("error out"=w398:errorcluster)  [unwired: 2 in, 3 out]
                n180 = call "_FPGA Set Digi Line.vi"("error in"=w398, "States"=w388, "Line (Set Latch1)"=_RW_Status."Set Latch3" ("Write Mode (Do Write)")) -> ("error out"=w396:errorcluster)  [unwired: 1 in, 3 out]
                n181 = call "_FPGA Set Digi Line.vi"("error in"=w396, "States"=w388, "Line (Set Latch1)"=_RW_Status."Set Latch4" ("Write Mode (Do Write)")) -> ("error out"=w387:errorcluster)  [unwired: 1 in, 3 out]
                n182 = Bundle By Name(cluster=w401, "Rt Loop Events"=RT_Loop_Events."Send Reply", "error"=w387) -> (w400:T10)
              }
              frame "Set Pol and DC" {
                w411 = "RT" ("section")
                # "Set Q1 POL, Q2 POL, Q1DC EN, Q2DC EN"
                n183 = Type Cast(type=u16 0, x=w425) -> (*(type *) &x=w420:u16)
                n184 = Number To Boolean Array(number=w420) -> (Boolean array=w419:bool[])
                n185 = call "_FPGA Set Digi Line.vi"("States"=w420, "Line (Set Latch1)"=_RW_Status."Set Latch1" ("Write Mode (Do Write)")) -> ("error out"=w407:errorcluster)  [unwired: 2 in, 3 out]
                n186 = Index Array(array=w419) -> (element #1=w409:bool, element #2=w408:bool)  [unwired: 2 in]
                n187 = global write "_RT Global.vi" "Q1 POL"(w409) -> ()
                n188 = global write "_RT Global.vi" "Q2 POL"(w408) -> ()
                n189 = call "_RT Open Preference File.vi"("error In"=w407) -> ("error"=w416:errorcluster, "refnum"=w415:T21)  [unwired: 5 out]
                n190 = call-poly <vilib>:"Write Key.vi"("section"=w411, "error in (no error)"=w416, "value"=w409, "key"="Q1Pol", "refnum"=w415) -> ("error out"=w413:errorcluster, "refnum out"=w412:T21)  [unwired: 5 out]
                n191 = call-poly <vilib>:"Write Key.vi"("section"=w411, "error in (no error)"=w413, "value"=w408, "key"="Q2Pol", "refnum"=w412) -> ("error out"=w418:errorcluster, "refnum out"=w417:T21)  [unwired: 5 out]
                n192 = call <vilib>:"Close Config Data.vi"("error in (no error)"=w418, "refnum"=w417) -> ("error out"=w406:errorcluster)  [unwired: 1 in, 8 out]
                n193 = Bundle By Name(cluster=w422, "Rt Loop Events"=RT_Loop_Events."Send Reply", "error"=w406) -> (w421:T10)
              }
              frame "Toggle RP" {
                # "Toggle Roughing Pump"
                n194 = Not Equal?(x=w429, y="0") -> (x != y?=w430:bool)
                n195 = Boolean To (0,1)(Boolean=w430) -> (0, 1=w428:i16)
                n196 = call "_FPGA Set Digi Line.vi"("States"=w428, "Line (Set Latch1)"=_RW_Status."RP ON" ("Write Mode (Do Write)")) -> ("error out"=w427:errorcluster)  [unwired: 2 in, 3 out]
                n197 = Bundle By Name(cluster=w433, "Rt Loop Events"=RT_Loop_Events."Send Reply", "error"=w427) -> (w432:T10)
              }
              frame "Toggle EL" {
                # "Toggle Electrics"
                n198 = Not Equal?(x=w440, y="0") -> (x != y?=w438:bool)
                n199 = Boolean To (0,1)(Boolean=w438) -> (0, 1=w437:i16)
                n200 = call "_FPGA Toggle Electronics.vi"("Ele On (1 for ON and 0 for OFF)"=w437) -> ("error out"=w436:errorcluster)  [unwired: 2 in, 5 out]
                n201 = Bundle By Name(cluster=w442, "Rt Loop Events"=RT_Loop_Events."Send Reply", "error"=w436) -> (w441:T10)
              }
              frame "Set PIC" {
                # "Set PIC"
                n202 = xnode "Read/Write Control"("FPGA VI Reference In"=w451) -> ("error out"=w450:errorcluster, "Running"=w447:bool)  [unwired: 1 in, 1 out]
                n203 = Unflatten From String(type=u32[] [], binary string=w455) -> (value=w449:u32[])  [unwired: 1 in, 4 out]
                n204 = local write "Running"(w447) -> ()
                n205 = case shown="False" w447 {
                  tunnel: w450 -> [w461 w463]
                  tunnel: w449 -> [w459 _]
                  tunnel: [w460 w462] -> w446
                  tunnel: [w456 _] -> w445
                  frame False {
                    n206 = Index Array(array=w459) -> (element #1=w458:u32, element #2=w457:u32)  [unwired: 2 in]
                    n207 = call "_FPGA Set PIC.vi"("error in"=w461, "Param 2"=w457, "Param 1"=w458) -> ("error out"=w460:errorcluster, "Data"=w456:u32)  [unwired: 2 in, 1 out]
                  }
                  frame True {
                    n208 = call "_Construct Error Cluster.vi"("error in"=w463, "reason"="Cannot send command to PIC because the instrument is busy.") -> ("error out"=w462:errorcluster)  [unwired: 2 in, 3 out]
                  }
                }
                n209 = Build Array(w445) -> (w444:u32[])
                n210 = Bundle By Name(cluster=w453, "Rt Loop Events"=RT_Loop_Events."Send Reply", "Data Array"=w444, "error"=w446) -> (w452:T10)
              }
              frame "P1" {
                # "Set COR POL, CUR POL for Latch2"
                n211 = Type Cast(type=u16 0, x=w471) -> (*(type *) &x=w465:u16)
                n212 = call "_FPGA Set Digi Line.vi"("States"=w465, "Line (Set Latch1)"=_RW_Status."Set Latch2" ("Write Mode (Do Write)")) -> ("error out"=w466:errorcluster)  [unwired: 2 in, 3 out]
                n213 = Bundle By Name(cluster=w468, "Rt Loop Events"=RT_Loop_Events."Send Reply", "error"=w466) -> (w467:T10)
              }
              frame "P2" {
                # "Set S1 POL, S2 POL for Latch3"
                n214 = Type Cast(type=u16 0, x=w479) -> (*(type *) &x=w473:u16)
                n215 = call "_FPGA Set Digi Line.vi"("States"=w473, "Line (Set Latch1)"=_RW_Status."Set Latch3" ("Write Mode (Do Write)")) -> ("error out"=w474:errorcluster)  [unwired: 2 in, 3 out]
                n216 = Bundle By Name(cluster=w476, "Rt Loop Events"=RT_Loop_Events."Send Reply", "error"=w474) -> (w475:T10)
              }
              frame "P3" {
                # "Set CEM POL for Latch4"
                n217 = Type Cast(type=u16 0, x=w487) -> (*(type *) &x=w481:u16)
                n218 = call "_FPGA Set Digi Line.vi"("States"=w481, "Line (Set Latch1)"=_RW_Status."Set Latch4" ("Write Mode (Do Write)")) -> ("error out"=w482:errorcluster)  [unwired: 2 in, 3 out]
                n219 = Bundle By Name(cluster=w484, "Rt Loop Events"=RT_Loop_Events."Send Reply", "error"=w482) -> (w483:T10)
              }
              frame "Send Serial" {
                # "Send Serial Command"
                n220 = Unflatten From String(type=T13 {"Port Type"=0, "baud rate (9600)"=9600, "data bits (8)"=8, "stop bits (1)"=10, "parity (0:none)"=0, "DoRead"=FALSE, "Command"=""} ("Serial Command"), binary string=w499) -> (value=w493:T13)  [unwired: 1 in, 4 out]
                n221 = xnode "Read/Write Control"("FPGA VI Reference In"=w495) -> ("error out"=w494:errorcluster, "Running"=w492:bool)  [unwired: 1 in, 1 out]
                n222 = local write "Running"(w492) -> ()
                n223 = case shown="False" w492 {
                  tunnel: w494 -> [w502 w505]
                  tunnel: w493 -> [w501 _]
                  tunnel: [w503 w504] -> w491
                  tunnel: [w500 _] -> w489
                  frame False {
                    n224 = call "_FPGA Send Serial.vi"("error in"=w502, "Serial Command"=w501) -> ("error out"=w503:errorcluster, "Reply"=w500:string)  [unwired: 2 in, 2 out]
                  }
                  frame True {
                    n225 = call "_Construct Error Cluster.vi"("error in"=w505, "reason"="Cannot send command to serial port because the instrument is busy.") -> ("error out"=w504:errorcluster)  [unwired: 2 in, 3 out]
                  }
                }
                n226 = Bundle By Name(cluster=w497, "Rt Loop Events"=RT_Loop_Events."Send Reply", "Message Data"=w489, "error"=w491) -> (w496:T10)
              }
              frame "Set LC Out" {
                # "Set LC Outputs"
                n227 = Type Cast(type=u16 0, x=w509) -> (*(type *) &x=w508:u16)
                n228 = call "_FPGA Write Data.vi"("Write Mode (Do Write)"=_RW_Status."Set LC Out", "Address"=w508) -> ("error out"=w507:errorcluster)  [unwired: 4 in, 2 out]
                n229 = Bundle By Name(cluster=w513, "Rt Loop Events"=RT_Loop_Events."Send Reply", "error"=w507) -> (w512:T10)
              }
              frame "Get LC In" {
                # "Get LC Inputs"
                n230 = call "_FPGA Read Data.vi"("Read Mode (Do Read)"=_RW_Status."Get LC In" ("R/W Status")) -> ("error out"=w515:errorcluster, "Data"=w516:u32)  [unwired: 4 in, 1 out]
                n231 = Split Number(x=w516) -> (hi(x)=w520:u16, lo(x)=w519:u16)
                n232 = Build Array(w520, w519) -> (w518:u16[])
                n233 = Bundle By Name(cluster=w522, "Rt Loop Events"=RT_Loop_Events."Send Reply", "Data Array"=w518, "error"=w515) -> (w521:T10)
              }
              frame "Read VAC" {
                # "Read VAC Gauge"
                n234 = call "_FPGA Read Data.vi"("Read Mode (Do Read)"=_RW_Status."Read VAC" ("R/W Status")) -> ("error out"=w524:errorcluster, "Data"=w525:u32)  [unwired: 4 in, 1 out]
                n235 = Build Array(w525) -> (w527:u32[])
                n236 = Bundle By Name(cluster=w529, "Rt Loop Events"=RT_Loop_Events."Send Reply", "Data Array"=w527, "error"=w524) -> (w528:T10)
              }
              frame "Test Table" {
                w542 = u16 405 ("Address")
                # "Run Table Test"
                n237 = Unflatten From String(type=u32[] [], binary string=w546) -> (value=w545:u32[])  [unwired: 1 in, 4 out]
                n238 = Index Array(array=w545) -> (element #1=w544:u32, element #2=w541:u32)  [unwired: 2 in]
                n239 = call "_FPGA Write Data.vi"("Data"=w544, "Address"=w542) -> ("error out"=w543:errorcluster)  [unwired: 4 in, 2 out]
                n240 = Increment(x=w542) -> (x+1=w539:u16)
                n241 = call "_FPGA Write Data.vi"("error in"=w543, "Data"=w541, "Address"=w539) -> ("error out"=w540:errorcluster)  [unwired: 3 in, 2 out]
                n242 = xnode "Read/Write Control"("FPGA VI Reference In"=w531, "error in"=w540, "R/W Status"=_RW_Status."Table Test") -> ("FPGA VI Reference Out"=w550:T11, "error out"=w549:errorcluster)
                n243 = xnode "Read/Write Control"("FPGA VI Reference In"=w550, "error in"=w549, "Read/Write"=TRUE ("Data Written")) -> ("error out"=w551:errorcluster)  [unwired: 1 out]
                n244 = Increment(x=w539) -> (x+1=w535:u16)
                n245 = call "_FPGA Wait Done.vi"("error in"=w551, "Indicator"=_FPGA_Indicator."Done") -> ("error out"=w538:errorcluster)  [unwired: 3 in, 2 out]
                n246 = Increment(x=w535) -> (x+1=w536:u16)
                n247 = call "_FPGA Read Data.vi"("error in"=w538, "Address"=w535) -> ("error out"=w537:errorcluster, "Data"=w533:u32)  [unwired: 3 in, 1 out]
                n248 = call "_FPGA Read Data.vi"("error in"=w537, "Address"=w536) -> ("error out"=w534:errorcluster, "Data"=w532:u32)  [unwired: 3 in, 1 out]
                n249 = Build Array(w533, w532) -> (w548:u32[])
                n250 = Bundle By Name(cluster=w556, "Rt Loop Events"=RT_Loop_Events."Send Reply", "Data Array"=w548, "error"=w534) -> (w555:T10)
              }
              frame "Toggle Power" {
                w571 = u8 0 ("default (0 I32)")
                # "Toggle the startup/shut down"
                n251 = call <vilib>:"Trim Whitespace.vi"("string"=w574) -> ("trimmed string"=w573:string)  [unwired: 1 in]
                n252 = global read "_RT Global.vi" "InstrState"() -> (w560:T3)
                n253 = Decimal String To Number(string=w573, default (0L)=w571) -> (number=w572:u8)  [unwired: 2 out]
                n254 = In Range and Coerce(upper limit=u8 2, x=w572, lower limit=w571) -> (coerced(x)=w564:u8)  [unwired: 1 out]
                n255 = Not Equal?(x=w560, y=_RT_Instrument_State."Starting Up") -> (x != y?=w566:bool)
                n256 = Not Equal?(x=w560, y=_RT_Instrument_State."Turbo Startup") -> (x != y?=w561:bool)
                n257 = Not Equal?(x=w560, y=_RT_Instrument_State."Shutting Down") -> (x != y?=w558:bool)
                n258 = Not Equal?(x=w564, y=u8 1) -> (x != y?=w565:bool)
                n259 = Compound Arithmetic op=AND(w566, w561, w558) -> (w562:bool)
                n260 = Or(x=w565, y=w562) -> (x .or. y?=w563:bool)
                n261 = case shown="True" w563 {
                  tunnel: w564 -> [_ w579]
                  frame False {
                  }
                  frame True {
                    n262 = Greater Than 0?(x=w579) -> (x > 0?=w578:bool)
                    n263 = global write "_RT Global.vi" "StartupMode"(w579) -> ()
                    n264 = case shown="True" w578 {
                      frame False {
                      }
                      frame True {
                        n265 = call "_FPGA Turn LC Pump Off.vi"() -> ()  [unwired: 2 in]
                      }
                    }
                  }
                }
                n266 = Bundle By Name(cluster=w577, "Rt Loop Events"=RT_Loop_Events."Send Reply") -> (w576:T10)
              }
              frame "Get Startup" {
                # "Get Startup Options"
                n267 = global read "_RT Global.vi" "StartupOptions"() -> (w581:T18)
                n268 = Flatten To String(anything=w581) -> (data string=w580:string)  [unwired: 1 in, 4 out]
                n269 = Bundle By Name(cluster=w583, "Rt Loop Events"=RT_Loop_Events."Send Reply", "Message Data"=w580) -> (w582:T10)
              }
              frame "Set Startup" {
                # "Set Startup Options"
                n270 = global read "_RT Global.vi" "StartupOptions"() -> (w595:T18)
                n271 = Unflatten From String(type=w595, binary string=w587) -> (value=w594:T18, error out=w586:errorcluster)  [unwired: 1 in, 3 out]
                n272 = global write "_RT Global.vi" "StartupOptions"(w594) -> ()
                n273 = call "_RT Open Preference File.vi"("error In"=w586) -> ("error"=w593:errorcluster, "refnum"=w592:T21)  [unwired: 5 out]
                n274 = call-poly <vilib>:"Write Key.vi"("section"="RT", "error in (no error)"=w593, "value"=w587, "key"="SUOpt", "refnum"=w592) -> ("error out"=w588:errorcluster, "refnum out"=w589:T21)  [unwired: 1 in, 4 out]
                n275 = call <vilib>:"Close Config Data.vi"("error in (no error)"=w588, "refnum"=w589) -> ("error out"=w585:errorcluster)  [unwired: 1 in, 8 out]
                n276 = Bundle By Name(cluster=w597, "Rt Loop Events"=RT_Loop_Events."Send Reply", "error"=w585) -> (w596:T10)
              }
              frame "Get ADC Table" {
                # "Get ADC Table"
                n277 = global read "_RT Global.vi" "ADC Table"() -> (w600:T20[])
                n278 = Flatten To String(anything=w600) -> (data string=w599:string)  [unwired: 1 in, 4 out]
                n279 = Bundle By Name(cluster=w603, "Rt Loop Events"=RT_Loop_Events."Send Reply", "Message Data"=w599) -> (w602:T10)
              }
              frame "Set ADC Table" {
                # "Set ADC Table"
                n280 = global read "_RT Global.vi" "ADC Table"() -> (w614:T20[])
                n281 = Unflatten From String(type=w614, binary string=w615) -> (value=w610:T20[], error out=w607:errorcluster)  [unwired: 1 in, 3 out]
                n282 = call "_Get Startup File.vi"("FileName"="ADC" ("key")) -> ("FilePath"=w605:path)
                n283 = global write "_RT Global.vi" "ADC Table"(w610) -> ()
                n284 = Write to Binary File(file (use dialog)=w605, data=w610, error in=w607) -> (refnum out=w608:refnum<file>, error out=w609:errorcluster)  [unwired: 4 out]
                n285 = Close File(refnum=w608, error in=w609) -> (error out=w606:errorcluster)  [unwired: 1 out]
                n286 = Bundle By Name(cluster=w612, "Rt Loop Events"=RT_Loop_Events."Send Reply", "error"=w606) -> (w611:T10)
              }
              frame "Get Brief Status" {
                # "#AK: modified the condition to send the logs to be always active"
                # "Get Brief Instrument Status Report"
                n287 = Empty String/Path?(string/path=w622) -> ()  [unwired: 1 out]
                n288 = local read "Running"() -> (w617:bool)
                n289 = global read "_RT Global.vi" "ADC Values"() -> (w620:i32[])
                n290 = call "_Calculate ADC Value.vi"("ADC Values"=w620, "ADC Channel (64)"=u8 64) -> ("User Value"=w627:sgl, "In Range?"=w619:bool)  [unwired: 1 out]
                n291 = call "_Calculate ADC Value.vi"("ADC Values"=w620, "ADC Channel (64)"=u8 72) -> ("In Range?"=w618:bool)  [unwired: 2 out]
                n292 = for {
                  tunnel: i32[] [119, 113, 114, 110, 108, 105, 120, 72, 71, 65, 67, 66, 68, 106, 107, 109] -> [w648] mode=indexing
                  tunnel: w620 -> [w649]
                  tunnel: [w647] -> w634 mode=indexing
                  tunnel: [w646] -> w636 mode=indexing
                  n293 = call "_Calculate ADC Value.vi"("ADC Values"=w649, "ADC Channel (64)"=w648) -> ("User Value"=w647:sgl, "In Range?"=w646:bool)  [unwired: 1 out]
                }
                n294 = case shown="False" w617 {
                  tunnel: [w641 830 ("Speed")] -> w629
                  frame False {
                    n295 = call "_FPGA Turbo Control.vi"("Command"=_Pump_Parameter."Read Actual Rotation Speed in Hz") -> ("Speed"=w641:i32)  [unwired: 3 in, 5 out]
                  }
                  frame True {
                  }
                }
                n296 = Build Array (concatenate)(w634, w627, w629) -> (w630:sgl[])
                n297 = Greater Or Equal?(x=w629, y=830) -> (x >= y?=w631:bool)
                n298 = Build Array (concatenate)(w636, w619, w631, w618) -> (w632:bool[])
                n299 = Flatten To String(anything=w630) -> (data string=w624:string)  [unwired: 1 in, 4 out]
                n300 = Boolean To (0,1)(Boolean=w632) -> (0, 1=w635:i16[])
                n301 = case shown="True" TRUE {
                  tunnel: [_ w644] -> w626
                  frame False {
                    # "for Server"
                  }
                  frame True {
                    # "Ion Sniffer"
                    n302 = call "_RT Event.vi"("Action (Write)"=enum16{"Write", "Read"}."Read") -> ("Log"=w644:string)  [unwired: 2 in, 4 out]
                  }
                }
                n303 = Format Into String(format string="%s<RTLog>%s", w624, w626) -> (resulting string=w623:string)  [unwired: 2 in, 1 out]
                n304 = Bundle By Name(cluster=w639, "Rt Loop Events"=RT_Loop_Events."Send Reply", "Data Array"=w635, "Message Data"=w623) -> (w638:T10)
              }
              frame "xml System Status", "Get Detail Status" {
                # "Get Detailed Instrument Status Report"
                n305 = global read "_RT Global.vi" "StartupOptions"() -> (w653:T18)
                n306 = xnode "Read/Write Control"("FPGA VI Reference In"=w656) -> ("Acquiring Data"=w660:bool, "Ready to Acquire Data"=w659:bool, "Running"=w658:bool)  [unwired: 1 in, 2 out]
                n307 = global read "_RT Global.vi" "Exhaust gas error"() -> (w651:bool)
                n308 = Unbundle By Name(w653) -> ("SourceExhaust"=w652:bool)
                n309 = And(x=w651, y=w652) -> (x .and. y?=w650:bool)
                n310 = local read "Fault"() -> (w655:bool)
                n311 = local read "Ready"() -> (w661:bool)
                n312 = local write "Running"(w658) -> ()
                n313 = Or(x=w650, y=w655) -> (x .or. y?=w654:bool)
                n314 = Select(t="4", s=w659, f="0") -> (s? t:f=w667:string)
                n315 = Select(t="1", s=w660, f=w667) -> (s? t:f=w669:string)
                n316 = Select(t=w669, s=w661, f="2") -> (s? t:f=w664:string)
                n317 = Select(t="3", s=w654, f=w664) -> (s? t:f=w657:string)
                n318 = call "_FPGA Get System Status.vi"("Server State"=w657) -> ("Status"=w670:string)  [unwired: 1 in, 5 out]
                n319 = Bundle By Name(cluster=w672, "Rt Loop Events"=RT_Loop_Events."Send Reply", "Message Data"=w670) -> (w671:T10)
              }
              frame "Auxiliary Update" {
                # "Send auxiliary update command"
                n320 = Scan From String(format string="%d,%f", input string=w678, default 1=-1 ("default value 1"), default 2=sgl 0.0 ("default value 2")) -> (output 1=w677:i32, output 2=w676:sgl)  [unwired: 2 in, 3 out]
                n321 = call "_FPGA Auxiliary Update.vi"("Setting Value"=w676, "Command Type"=w677) -> ("error out"=w675:errorcluster, "Return Value"=w674:string)  [unwired: 1 in, 3 out]
                n322 = Bundle By Name(cluster=w683, "Rt Loop Events"=RT_Loop_Events."Send Reply", "Message Data"=w674, "error"=w675) -> (w682:T10)
              }
              frame "Set CC Logics" {
                # "Set contact closure output logics:\n0 for Shimadzu; 1 for others"
                n323 = Type Cast(type=u16 0, x=w689) -> (*(type *) &x=w686:u16)
                n324 = call "_FPGA Write Data.vi"("Write Mode (Do Write)"=_RW_Status."Do Write", "Data"=w686, "Address"=u16 399) -> ("error out"=w685:errorcluster)  [unwired: 3 in, 2 out]
                n325 = Bundle By Name(cluster=w692, "Rt Loop Events"=RT_Loop_Events."Send Reply", "error"=w685) -> (w691:T10)
              }
              frame "xml Set LC Input Logic", "Set CC Input Logics" {
                # "Set contact closure input logics:\nOption    LC1        LC2\n     0        High      High\n     1        Low        High\n     2        High       Low\n     3        Low        Low"
                n326 = case shown="\"xml Set LC Input Logic\", Default" w694 {
                  tunnel: w699 -> [w705 w707]
                  tunnel: [w703 w706] -> w696
                  frame "xml Set LC Input Logic", Default {
                    n327 = Unflatten From String(type=u16 0, binary string=w705) -> (value=w703:u16)  [unwired: 3 in, 2 out]
                  }
                  frame "Set CC Input Logics" {
                    n328 = Type Cast(type=u16 0, x=w707) -> (*(type *) &x=w706:u16)
                  }
                }
                n329 = call "_FPGA Write Data.vi"("Write Mode (Do Write)"=_RW_Status."Do Write", "Data"=w696, "Address"=u16 409) -> ("error out"=w695:errorcluster)  [unwired: 3 in, 2 out]
                n330 = Bundle By Name(cluster=w701, "Rt Loop Events"=RT_Loop_Events."Send Reply", "error"=w695) -> (w700:T10)
              }
              frame "Ignore Error" {
                # "Set Igore Lost Communication Error Flag\n0 = false\n1 = true (ignore error)"
                n331 = call <vilib>:"Trim Whitespace.vi"("string"=w712) -> ("trimmed string"=w711:string)  [unwired: 1 in]
                n332 = Not Equal?(x=w711, y="0") -> (x != y?=w709:bool)
                n333 = global write "_RT Global.vi" "IgnoreError"(w709) -> ()
                n334 = Bundle By Name(cluster=w715, "Rt Loop Events"=RT_Loop_Events."Send Reply") -> (w714:T10)
              }
              frame "Set Max Mass" {
                # "Set Maximum Mass"
                n335 = global read "_RT Global.vi" "Max Mass"() -> (w720:dbl)
                n336 = Unflatten From String(type=w720, binary string=w721) -> (error out=w716:errorcluster)  [unwired: 1 in, 4 out]
                n337 = Bundle By Name(cluster=w718, "Rt Loop Events"=RT_Loop_Events."Send Reply", "error"=w716) -> (w717:T10)
              }
              frame Default {
                n338 = Format Into String(format string="Message Type: %s, not recognized by firmware command receiver.", w722) -> (resulting string=w727:string)  [unwired: 2 in, 1 out]
                n339 = call "_Construct Error Cluster.vi"("reason"=w727) -> ("error out"=w723:errorcluster)  [unwired: 3 in, 3 out]
                n340 = Bundle By Name(cluster=w725, "Rt Loop Events"=RT_Loop_Events."Send Reply", "error"=w723) -> (w724:T10)
              }
            }
          }
          frame True {
            # "No command received from the host at this time,\nor the host has been disconnected."
            n341 = case shown="7100.., Default" w730 {
              tunnel: w733 -> [w737 w745]
              tunnel: [w736 w744] -> w732
              tunnel: w731 -> [_ w741]
              tunnel: w729 -> [w735 _]
              frame 7100.., Default {
                n342 = Bundle By Name(cluster=w737, "error"=w735, "Rt Loop Events"=RT_Loop_Events."Send Reply") -> (w736:T10)
              }
              frame 56, 59, 62, 64, 66 {
                n343 = local read "# Connections"() -> (w742:u8)
                n344 = Greater?(x=w742, y=u8 2) -> (0:w739:bool)
                n345 = case shown="True" w739 {
                  tunnel: w742 -> [w748 _]
                  tunnel: w741 -> [_ w751]
                  tunnel: [RT_Loop_Events."Wait for Command" ("Rt Loop Events") RT_Loop_Events."Wait for Connection" ("Rt Loop Events")] -> w740
                  frame False {
                    n346 = Increment(x=w748) -> (x+1=w746:u8)
                    n347 = local write "# Connections"(w746) -> ()
                  }
                  frame True {
                    n348 = TCP Close Connection(connection ID=w751, abort (F)=TRUE) -> ()  [unwired: 1 in, 2 out]
                    "Connected?" <- FALSE ("Connected?")
                  }
                }
                n349 = Wait Until Next ms Multiple(millisecond multiple=u32 380 ("milliseconds to wait")) -> ()  [unwired: 1 out]
                n350 = Bundle By Name(cluster=w745, "Rt Loop Events"=w740) -> (w744:T10)
              }
            }
          }
        }
      }
      frame "Send Reply" {
        w770 = i32[] []  # Data Array
        w769 = errorcluster {"status"=FALSE, "code"=0, "source"=""}  # error
        w771 = ""  # Info
        # "Send a reply back to the host after receiving each command"
        n351 = Unbundle By Name(w758) -> ("Connection ID"=w774:refnum<k5>, "error"=w765:errorcluster, "Sequence Number"=w764:i32, "Command"=w763:T1, "Message Data"=w762:string, "error"=w761:errorcluster, "Data Array"=w759:i32[])
        n352 = case shown="\"xml Start Run\"..\"xml Get Info\"" w763 {
          selector: w763 -> [w776 w783]
          tunnel: w762 -> [w781 w785]
          tunnel: w761 -> [w780 w784]
          tunnel: [w778 w785] -> w756
          tunnel: [w775 w784] -> w760
          tunnel: w759 -> [w779 _]
          tunnel: [w776 w783] -> w757
          frame Default {
            n353 = Bundle By Name(cluster=T17 {"Info"="", "Data Array"=[], "error out"={"status"=FALSE, "code"=0, "source"=""}} ("Data"), "Info"=w781, "error out"=w780, "Data Array"=w779) -> (w777:T17)
            n354 = Flatten To String(anything=w777) -> (data string=w778:string, error out=w775:errorcluster)  [unwired: 3 in, 1 out]
          }
          frame "xml Start Run".."xml Get Info" {
          }
        }
        n355 = Bundle By Name(cluster=T16 {"Packet Signature"="", "Sequence Number"=0, "Command"=enum."Start", "Data Message Size"=0, "Data Message Size"="", "Data Message"="", "Error Message Size"=0, "Error Message Size"="", "Error Message"="", "Checksum"=0, "Error Message"={"status"=FALSE, "code"=0, "source"=""}, "Command ID"=""} ("Packet Info In"), "Sequence Number"=w764, "Command"=w757, "Data Message"=w756, "Error Message"=w760) -> (w766:T16)
        n356 = call "_TCP Msg Write.vi"("RT"=TRUE, "error in"=w765, "Packet Info In"=w766, "connection ID In"=w774) -> ()  [unwired: 1 in, 7 out]
        n357 = Bundle By Name(cluster=w758, "Rt Loop Events"=RT_Loop_Events."Wait for Command", "Message Data"=w771, "Data Array"=w770, "error"=w769) -> (w772:T10)
      }
    }
  }
  n358 = Get Date/Time In Seconds() -> (seconds since 1Jan1904=w12:timestamp)
  n359 = Tick Count (ms)() -> (millisecond timer value=w2:u32)
  n360 = To Double Precision Float(number=w12) -> (double precision float=w11:dbl)
  n361 = while {
    tunnel: w11 -> [w793]
    tunnel: w7 -> [_]
    tunnel: w1 -> [w786]
    shift-right: [w787] -> _
    shift-left: FALSE ("Connected?") -> [w790]
    stop <- FALSE stop-if-true
    n362 = Get Date/Time In Seconds() -> (seconds since 1Jan1904=w794:timestamp)
    n363 = To Double Precision Float(number=w794) -> (double precision float=w795:dbl)
    n364 = Subtract(x=w795, y=w793) -> (x-y=w796:dbl)
    "Time (s)" <- w796
    n365 = global write "_RT Global.vi" "RT Time(s)"(w796) -> ()
    n366 = local read "Connected?"() -> (w789:bool)
    n367 = Or(x=w790, y=w789) -> (x .or. y?=w788:bool)
    n368 = Select(t=u32 1800 ("milliseconds to wait"), s=w789, f=u32 280 ("milliseconds to wait")) -> (s? t:f=w801:u32)
    n369 = case shown="True" w788 {
      selector: w788 -> [w803 w804]
      tunnel: [w803 w804] -> w792
      tunnel: [0 ("State") 1 ("State")] -> w791
      frame False {
      }
      frame True {
      }
    }
    n370 = Wait (ms)(milliseconds to wait=w801) -> ()  [unwired: 1 out]
    n371 = Not(x=w792) -> (.not. x?=w787:bool)
    n372 = call <vilib>:"RT LEDs.vi"("error in (no error)"=w786, "State"=w791, "LED Num"=0) -> ()  [unwired: 3 in, 2 out]
  }
  n373 = while {
    tunnel: w7 -> [w810]
    shift-right: [w813] -> _
    shift-left: w10 -> [w812]
    shift-right: [w809] -> _
    shift-left: FALSE ("Key Pressed") -> [w808]
    shift-right: [w806] -> _
    shift-left: TRUE ("Key Pressed") -> [w807]
    stop <- FALSE stop-if-true
    n374 = case shown="\"Shutting Down\"" w812 {
      selector: w812 -> [_ w836 _ _ w866 _ _ _ w907 _ w941 w965 _ _ w1068 w1094 w1118 w1155 _ _]
      tunnel: w810 -> [_ _ _ _ _ _ _ _ _ _ _ _ w989 _ _ _ _ _ _ _]
      tunnel: [_RT_Instrument_State."Mass Spectrometer is Off" ("InstrState") w835 w840 _RT_Instrument_State."Roughing Pump Ready" ("InstrState") w867 w884 _RT_Instrument_State."Initializing" ("t") _RT_Instrument_State."Going to Standby" ("t") w906 _RT_Instrument_State."24V Standby" ("InstrState") w940 w964 w990 _RT_Instrument_State."Ready" ("InstrState") w1070 w1095 w1121 w1152 w1168 _RT_Instrument_State."Shutting Down" ("t")] -> w813
      tunnel: [w816 w830 w839 w845 w864 w881 w886 w893 w901 w925 w935 w963 w988 w1042 w1060 w1093 w1116 w1147 FALSE ("Key Pressed") w1177] -> w809
      tunnel: w808 -> [w816 _ w839 w845 w863 w881 w886 w893 w900 w925 w934 w962 w988 w1042 _ w1092 w1116 _ w1163 w1177]
      tunnel: w807 -> [w815 w829 w838 w844 w862 w880 w885 w892 w899 w924 w933 w961 _ w1041 w1059 w1091 w1115 w1146 w1158 w1176]
      tunnel: [w815 w829 w838 w844 w862 w880 w885 w892 w899 w924 w933 w961 w987 w1041 w1059 w1091 w1115 w1146 w1158 w1176] -> w806
      frame "Initializing" {
        w819 = T24 11 items=["Same", "Empty", "VacFail", "Cancel", "CheckGas", "EleFail", "Probe1Fail", "Probe2Fail", "HeaterFail", "DoorOpen", "CheckComm", "PressStart"] ("Line2Msg (same)")
        w820 = T25 2 items=["Same", "Empty", "Connected", "Starting", "Stopping", "Action", "On", "Service", "Call", "Acquiring", "Source"] ("Line1Msg (same)")
        w822 = FALSE ("Connected?")
        # "Going to System Off State"
        n375 = call "_FPGA Set LEDs.vi"("LED Command"=_LED_States."Off BRP") -> ("error out"=w824:errorcluster)  [unwired: 3 in, 3 out]
        n376 = Wait (ms)(milliseconds to wait=u32 1800) -> ()  [unwired: 1 out]
        n377 = call "_FPGA Set LCD Msg.vi"("error in"=w824, "Line2Msg (same)"=w819, "Line1Msg (same)"=w820) -> ("error out"=w817:errorcluster)  [unwired: 4 in, 2 out]
        n378 = call "_FPGA Send LCD.vi"("error in (no error)"=w817, "Command"=_RT_LED_Num."ReadKey" ("LED#")) -> ()  [unwired: 2 in, 5 out]
        n379 = global write "_RT Global.vi" "StartupMode"(u8 2 ("StartupMode")) -> ()
        n380 = local write "Running"(FALSE ("Connected?")) -> ()
        n381 = call "_RT Event.vi"("Event"="Mass Spectrometer is OFF. Power Connected") -> ()  [unwired: 2 in, 5 out]
        "Ready" <- w822
        "Fault" <- w822
      }
      frame "Mass Spectrometer is Off" {
        # "Wait for the start up command"
        n382 = call "_FPGA Read Key.vi"("CurStartupMode (0)"=u8 2, "ForStart (F)"=TRUE) -> ("Key Pressed"=w831:bool, "Key Pressed 2"=w830:bool)  [unwired: 2 in, 3 out]
        n383 = Select(t=_RT_Instrument_State."Starting Up", s=w831, f=w836) -> (s? t:f=w835:T3)
      }
      frame "Starting Up" {
        w842 = FALSE ("Status LED")
        # "Start a startup sequence"
        n384 = call "_FPGA Send LCD.vi"("Command"=_RT_LED_Num."ReadKey" ("LED#")) -> ("error out"=w841:errorcluster)  [unwired: 4 in, 3 out]
        n385 = call "_Update Start Up.vi"("error in (no error)"=w841) -> ("Next InstrState"=w840:T3)  [unwired: 2 in, 4 out]
        n386 = global write "_RT Global.vi" "Tuning Error Generated"(FALSE ("Tuning Error Generated")) -> ()
        n387 = local write "Ready"(w842) -> ()
        n388 = local write "Fault"(w842) -> ()
      }
      frame "Going to Standby" {
        w848 = T25 8 items=["Same", "Empty", "Connected", "Starting", "Stopping", "Action", "On", "Service", "Call", "Acquiring", "Source"] ("Line1Msg (same)")
        n389 = call "_FPGA Read ADC.vi"() -> ("error out"=w846:errorcluster)  [unwired: 3 in, 6 out]
        n390 = call "_FPGA Check Source ID.vi"("error in (no error)"=w846) -> ("Source ID OK"=w850:bool)
        n391 = call "_FPGA Set Parameters.vi"("ExhaustGas (on)"=FALSE, "error in"=w846, "HSID Temp (on)"=w850) -> ("error out"=w852:errorcluster)  [unwired: 6 in, 2 out]
        n392 = call "_FPGA Set LEDs.vi"("error in (no error)"=w852, "LED Command"=_LED_States."Off BRP") -> ("error out"=w851:errorcluster)  [unwired: 2 in, 3 out]
        n393 = call "_FPGA Set LEDs.vi"("error in (no error)"=w851, "LED Command"=_LED_States."Solid P") -> ("error out"=w856:errorcluster)  [unwired: 2 in, 3 out]
        n394 = call "_FPGA Set LCD Msg.vi"("error in"=w856, "Line1Msg (same)"=w848) -> ("error out"=w857:errorcluster)  [unwired: 5 in, 2 out]
        n395 = call "_RT Event.vi"("Event"="Roughing Pump Ready state.") -> ()  [unwired: 2 in, 5 out]
        n396 = call "_FPGA Send LCD.vi"("error in (no error)"=w857, "Command"=_RT_LED_Num."ReadKey" ("LED#")) -> ()  [unwired: 3 in, 4 out]
        n397 = global write "_RT Global.vi" "StartupMode"(u8 1 ("StartupMode")) -> ()
        n398 = disable-structure shown="Disabled" {
          frame Disabled {
            n399 = local write "Fault"(TRUE ("Fault")) -> ()
          }
          frame Enabled {
          }
        }
        n400 = local write "Ready"(FALSE ("Status LED")) -> ()
      }
      frame "Roughing Pump Ready" {
        n401 = global read "_RT Global.vi" "StartupMode"() -> (w865:u8)
        n402 = case shown="2" w865 {
          tunnel: [_RT_Instrument_State."Turbo Startup" ("InstrState") w875 _RT_Instrument_State."Shutting Down" ("InstrState")] -> w867
          tunnel: w866 -> [_ w873 _]
          tunnel: [w868 w870 w878] -> w864
          tunnel: w863 -> [w868 _ w878]
          frame 0 {
            # "Continue the startup sequence"
          }
          frame 1, Default {
            w872 = T25 11 items=["Same", "Empty", "Connected", "Starting", "Stopping", "Action", "On", "Service", "Call", "Acquiring", "Source", "Roughing Pump Ready"] ("Line1Msg (same)")
            # "Wait for Start key to restart the system"
            n403 = call "_FPGA Read Key.vi"("CurStartupMode (0)"=u8 1, "ForStart (F)"=TRUE) -> ("Key Pressed"=w871:bool, "Key Pressed 2"=w870:bool)  [unwired: 2 in, 3 out]
            n404 = call "_FPGA Set LCD Msg.vi"("Line1Msg (same)"=w872) -> ()  [unwired: 8 in, 1 out]
            n405 = Select(t=_RT_Instrument_State."Turbo Startup", s=w871, f=w873) -> (s? t:f=w875:T3)
          }
          frame 2 {
            # "Received a shutdown command"
          }
        }
      }
      frame "Turbo Startup" {
        # "Continue the startup sequence"
        n406 = call "_FPGA Send LCD.vi"("Command"=_RT_LED_Num."ReadKey" ("LED#")) -> ("error out"=w882:errorcluster)  [unwired: 4 in, 3 out]
        n407 = call "_Update Start Up Turbo.vi"("error in (no error)"=w882) -> ("Next InstrState"=w884:T3)  [unwired: 2 in, 4 out]
      }
      frame "Turning Power Off" {
        w887 = T25 4 items=["Same", "Empty", "Connected", "Starting", "Stopping", "Action", "On", "Service", "Call", "Acquiring", "Source"] ("Line1Msg (same)")
        n408 = call "_FPGA Set LCD Msg.vi"("Line1Msg (same)"=w887) -> ()  [unwired: 6 in, 3 out]
        n409 = local write "Ready"(FALSE ("Status LED")) -> ()
        n410 = local write "Fault"(TRUE ("Status LED")) -> ()
        n411 = Wait (ms)(milliseconds to wait=u32 1800) -> ()  [unwired: 1 out]
      }
      frame "Turning Turbo Off" {
        n412 = stacked-sequence {
          frame #0 {
            n413 = Wait (ms)(milliseconds to wait=u32 1800) -> ()  [unwired: 1 out]
          }
          frame #1 {
            n414 = call "_FPGA Send LCD.vi"("Command"=_RT_LED_Num."ReadKey" ("LED#")) -> ()  [unwired: 4 in, 4 out]
          }
        }
        n415 = local write "Ready"(FALSE ("Status LED")) -> ()
        n416 = local write "Fault"(TRUE ("Status LED")) -> ()
      }
      frame "Turbopump Ready" {
        w903 = T25 5 items=["Same", "Empty", "Connected", "Starting", "Stopping", "Action", "On", "Service", "Call", "Acquiring", "Source"] ("Line1Msg (same)")
        n417 = global read "_RT Global.vi" "StartupMode"() -> (w908:u8)
        n418 = local write "Fault"(TRUE ("Status LED")) -> ()
        n419 = call "_FPGA Set LCD Msg.vi"("Line1Msg (same)"=w903) -> ("error out"=w902:errorcluster)  [unwired: 6 in, 2 out]
        n420 = case shown="Default" w908 {
          tunnel: [w918 _RT_Instrument_State."Shutting Down" ("InstrState") _RT_Instrument_State."Checking Vacuum" ("InstrState")] -> w906
          tunnel: w907 -> [w915 _ _]
          tunnel: w902 -> [_ _ _]
          tunnel: [w910 w920 w922] -> w901
          tunnel: w900 -> [_ w920 w922]
          frame Default {
            # "Allow system to shut down from this state"
            n421 = local read "Connected?"() -> (w917:bool)
            n422 = call "_FPGA Read Key.vi"("CurStartupMode (0)"=u8 1) -> ("error out"=w912:errorcluster, "Key Pressed"=w911:bool, "Key Pressed 2"=w910:bool)  [unwired: 3 in, 2 out]
            n423 = call "_FPGA System Polling.vi"("error in (no error)"=w912, "Connected?"=w917, "CurInstrState"=w915, "High Vac Reached?"=TRUE) -> ("Running"=w916:bool, "Next InstrState"=w914:T3)  [unwired: 1 in, 2 out]
            n424 = local write "Running"(w916) -> ()
            n425 = Select(t=_RT_Instrument_State."Shutting Down", s=w911, f=w914) -> (s? t:f=w918:T3)
          }
          frame 2 {
            # "Received a shutdown command"
          }
          frame 0 {
            # "Received a startup command"
          }
        }
        n426 = local write "Ready"(FALSE ("Status LED")) -> ()
      }
      frame "Go to 24V Standby" {
        w929 = T25 7 items=["Same", "Empty", "Connected", "Starting", "Stopping", "Action", "On", "Service", "Call", "Acquiring", "Source"] ("Line1Msg (same)")
        n427 = local write "Fault"(TRUE ("Status LED")) -> ()
        n428 = call "_FPGA Set LCD Msg.vi"("Line1Msg (same)"=w929) -> ("error out"=w926:errorcluster)  [unwired: 6 in, 2 out]
        n429 = global read "_RT Global.vi" "Ele On"() -> (w928:bool)
        n430 = local write "Ready"(FALSE ("Status LED")) -> ()
        n431 = case shown="True" w928 {
          tunnel: w926 -> [_ _]
          frame False {
          }
          frame True {
            # "Turn off electronics"
            n432 = call "_FPGA Toggle Electronics.vi"() -> ()  [unwired: 3 in, 6 out]
          }
        }
        n433 = call "_RT Event.vi"("Event"="Going to 24V Standby state.") -> ()  [unwired: 2 in, 5 out]
      }
      frame "Turbopump Ready-Waiting" {
        w937 = T25 8 items=["Same", "Empty", "Connected", "Starting", "Stopping", "Action", "On", "Service", "Call", "Acquiring", "Source"] ("Line1Msg (same)")
        n434 = global read "_RT Global.vi" "StartupMode"() -> (w942:u8)
        n435 = local write "Fault"(TRUE ("Status LED")) -> ()
        n436 = call "_FPGA Set LCD Msg.vi"("Line1Msg (same)"=w937) -> ("error out"=w936:errorcluster)  [unwired: 6 in, 2 out]
        n437 = case shown="Default" w942 {
          tunnel: [w949 _RT_Instrument_State."Shutting Down" ("InstrState") _RT_Instrument_State."Checking Vacuum" ("InstrState")] -> w940
          tunnel: w941 -> [w952 _ _]
          tunnel: w936 -> [_ _ _]
          tunnel: [w944 w957 w959] -> w935
          tunnel: w934 -> [_ w957 w959]
          tunnel: w933 -> [w943 _ _]
          frame Default {
            # "Allow system to proceed to ready from this state"
            n438 = local read "Connected?"() -> (w954:bool)
            n439 = call "_FPGA Read Key.vi"("CurStartupMode (0)"=u8 1, "ForStart (F)"=TRUE) -> ("error out"=w946:errorcluster, "Key Pressed"=w945:bool, "Key Pressed 2"=w944:bool)  [unwired: 2 in, 2 out]
            n440 = call "_FPGA System Polling.vi"("error in (no error)"=w946, "Waiting (F)"=TRUE, "Connected?"=w954, "CurInstrState"=w952, "High Vac Reached?"=w943) -> ("Running"=w953:bool, "Next InstrState"=w948:T3)  [unwired: 2 out]
            n441 = case shown="False" w945 {
              tunnel: [w955 _RT_Instrument_State."Checking Vacuum" ("t")] -> w949
              tunnel: w948 -> [w955 _]
              frame False {
              }
              frame True {
              }
            }
            n442 = local write "Running"(w953) -> ()
          }
          frame 2 {
            # "Received a shutdown command"
          }
          frame 0 {
            # "Received a startup command"
          }
        }
        n443 = local write "Ready"(FALSE ("Status LED")) -> ()
      }
      frame "24V Standby" {
        n444 = global read "_RT Global.vi" "StartupMode"() -> (w966:u8)
        n445 = case shown="2" w966 {
          tunnel: [w975 _RT_Instrument_State."Shutting Down" ("InstrState") _RT_Instrument_State."Starting Up" ("InstrState")] -> w964
          tunnel: w965 -> [w973 _ _]
          tunnel: [w968 w983 w985] -> w963
          tunnel: w962 -> [_ w983 w985]
          frame Default {
            w967 = TRUE ("Waiting (F)")
            # "Allow system to restart from this state"
            n446 = local read "Connected?"() -> (w979:bool)
            n447 = call "_FPGA Read Key.vi"("CurStartupMode (0)"=u8 1, "ForStart (F)"=TRUE) -> ("error out"=w970:errorcluster, "Key Pressed"=w969:bool, "Key Pressed 2"=w968:bool)  [unwired: 2 in, 2 out]
            n448 = call "_FPGA System Polling.vi"("error in (no error)"=w970, "Waiting (F)"=w967, "Connected?"=w979, "CurInstrState"=w973, "High Vac Reached?"=w967) -> ("Running"=w978:bool, "Next InstrState"=w974:T3)  [unwired: 2 out]
            n449 = Not Equal?(x=w973, y=w974) -> (x != y?=w972:bool)
            n450 = Or(x=w969, y=w972) -> (x .or. y?=w971:bool)
            n451 = case shown="False" w971 {
              tunnel: [w980 _RT_Instrument_State."Starting Up" ("t")] -> w975
              tunnel: w974 -> [w980 _]
              frame False {
              }
              frame True {
                n452 = global write "_RT Global.vi" "StartupMode"(u8 0 ("StartupMode")) -> ()
              }
            }
            n453 = local write "Running"(w978) -> ()
          }
          frame 2 {
            # "Received a shutdown command"
          }
          frame 0 {
            # "Received a startup command"
          }
        }
      }
      frame "Checking Vacuum" {
        n454 = stacked-sequence {
          seq-local: [w994 _] -> [_ w1014]
          seq-local: [w993 _] -> [_ w1013]
          seq-local: [w992 _] -> [_ w1012]
          tunnel: w989 -> [_ w1015]
          tunnel: [_ w1016] -> w990
          tunnel: [_ w1011] -> w987
          frame #0 {
            n455 = Tick Count (ms)() -> (millisecond timer value=w995:u32)
            n456 = call "_FPGA Set LEDs.vi"("LED Command"=_LED_States."Off BRP") -> ("error out"=w991:errorcluster)  [unwired: 3 in, 3 out]
            n457 = while {
              tunnel: w995 -> [w1007]
              tunnel: [w1006] -> w994
              tunnel: [w1004] -> w993
              tunnel: [w998] -> w992
              tunnel: w991 -> [_]
              stop <- w1000 stop-if-true
              w997 = u32 1800000  # 30min timeout
              n458 = Wait (ms)(milliseconds to wait=u32 800) -> (millisecond timer value=w1009:u32)
              n459 = Subtract(x=w1009, y=w1007) -> (x-y=w1002:u32)
              n460 = call "_Check Limit.vi"("Header"="Pumping 2:" ("Header (10Ch)"), "Current"=w1002, "Max (100)"=w997) -> ("Max Reached"=w1001:bool, "ProgressBar"=w999:string)  [unwired: 1 in, 2 out]
              n461 = call "_FPGA Check Vacuum.vi"() -> ("Vac OK"=w1006:bool, "Source OK"=w1004:bool, "Stop"=w1005:bool, "Shutdown"=w998:bool)  [unwired: 2 out]
              n462 = Or(x=w1005, y=w1001) -> (x .or. y?=w1000:bool)
              n463 = case shown="False" w1000 {
                tunnel: w999 -> [w1010 _]
                frame False {
                  n464 = call "_FPGA Set LCD Msg.vi"("Info"=w1010) -> ()  [unwired: 6 in, 3 out]
                }
                frame True {
                }
              }
            }
          }
          frame #1 {
            n465 = case shown="True" w1014 {
              tunnel: [w1020 w1036] -> w1016
              tunnel: w1015 -> [_ w1030]
              tunnel: w1013 -> [_ w1031]
              tunnel: w1012 -> [w1018 _]
              tunnel: [FALSE ("Key Pressed") TRUE ("Key Pressed")] -> w1011
              frame False {
                # "User aborted vacuum check or 30min timeout:\nHigh vacuum not achieved."
                n466 = case shown="False" w1018 {
                  tunnel: [_RT_Instrument_State."Turbopump Ready" ("t") _RT_Instrument_State."Shutting Down" ("t")] -> w1020
                  tunnel: [u8 1 ("StartupMode") u8 2 ("StartupMode")] -> w1019
                  frame False {
                    w1023 = T24 2 items=["Same", "Empty", "VacFail", "Cancel", "CheckGas", "EleFail", "Probe1Fail", "Probe2Fail", "HeaterFail", "DoorOpen", "CheckComm", "PressStart", "StartRP"] ("Line2Msg (same)")
                    w1024 = T25 5 items=["Same", "Empty", "Connected", "Starting", "Stopping", "Action", "On", "Service", "Call", "Acquiring", "Source"] ("Line1Msg (same)")
                    n467 = call "_RT Event.vi"("Event"="Going to Turbopump Ready state.") -> ()  [unwired: 2 in, 5 out]
                    n468 = call "_FPGA Set LCD Msg.vi"("ErrNum"="003", "Line2Msg (same)"=w1023, "Line1Msg (same)"=w1024) -> ()  [unwired: 4 in, 3 out]
                  }
                  frame True {
                  }
                }
                n469 = global write "_RT Global.vi" "StartupMode"(w1019) -> ()
              }
              frame True {
                # "High Vacuum Achieved"
                n470 = case shown="False" w1031 {
                  tunnel: [_RT_Instrument_State."Source Standby" ("t") _RT_Instrument_State."Going to Ready" ("t")] -> w1036
                  frame False {
                    n471 = call "_RT Event.vi"("Event"="Going to Source Standby state.") -> ()  [unwired: 2 in, 5 out]
                    n472 = global write "_RT Global.vi" "StartupMode"(u8 1 ("StartupMode")) -> ()
                  }
                  frame True {
                    # "Source OK"
                  }
                }
                n473 = xnode "Read/Write Control"("FPGA VI Reference In"=w1030, "FilaB"=FALSE) -> ("FPGA VI Reference Out"=w1033:T11, "error out"=w1034:errorcluster)  [unwired: 1 in]
                n474 = xnode "Read/Write Control"("FPGA VI Reference In"=w1033, "error in"=w1034, "FilaC"=TRUE) -> ()  [unwired: 2 out]
              }
            }
          }
        }
      }
      frame "Going to Ready" {
        w1046 = T24 1 items=["Same", "Empty", "VacFail", "Cancel", "CheckGas", "EleFail", "Probe1Fail", "Probe2Fail", "HeaterFail", "DoorOpen", "CheckComm", "PressStart", "StartRP"] ("Line2Msg (same)")
        w1047 = T25 6 items=["Same", "Empty", "Connected", "Starting", "Stopping", "Action", "On", "Service", "Call", "Acquiring", "Source"] ("Line1Msg (same)")
        n475 = call "_FPGA Set LEDs.vi"("LED Command"=_LED_States."Off BRP") -> ("error out"=w1049:errorcluster)  [unwired: 3 in, 3 out]
        n476 = call "_FPGA Set LEDs.vi"("error in (no error)"=w1049, "LED Command"=_LED_States."Solid P") -> ("error out"=w1051:errorcluster)  [unwired: 2 in, 3 out]
        n477 = call "_FPGA Set LCD Msg.vi"("error in"=w1051, "Line2Msg (same)"=w1046, "Line1Msg (same)"=w1047) -> ("error out"=w1054:errorcluster)  [unwired: 4 in, 2 out]
        n478 = call "_RT Event.vi"("Event"="Analyzer is Ready") -> ()  [unwired: 2 in, 5 out]
        n479 = call "_FPGA Send LCD.vi"("error in (no error)"=w1054, "Command"=_RT_LED_Num."ReadKey" ("LED#")) -> ("error out"=w1043:errorcluster)  [unwired: 3 in, 3 out]
        n480 = call "_FPGA Set Parameters.vi"("error in"=w1043, "Set Zero (on)"=FALSE) -> ()  [unwired: 7 in, 3 out]
        n481 = global write "_RT Global.vi" "StartupMode"(u8 0 ("StartupMode")) -> ()
        n482 = local write "Ready"(TRUE ("Status LED")) -> ()
        n483 = local write "Fault"(FALSE ("Status LED")) -> ()
      }
      frame "Ready", Default {
        n484 = local read "Connected?"() -> (w1069:bool)
        n485 = call "_FPGA Read Key.vi"() -> ("error out"=w1062:errorcluster, "Key Pressed"=w1061:bool, "Key Pressed 2"=w1060:bool)  [unwired: 4 in, 2 out]
        n486 = local read "RunMode"() -> (w1063:i32)
        n487 = call "_FPGA System Polling.vi"("error in (no error)"=w1062, "Connected?"=w1069, "CurInstrState"=w1068, "High Vac Reached?"=TRUE) -> ("Running"=w1064:bool, "Next InstrState"=w1067:T3)  [unwired: 1 in, 2 out]
        n488 = local write "Running"(w1064) -> ()
        n489 = case shown="3, 6, 7" w1063 {
          tunnel: [_ TRUE] -> w1066
          frame 0, Default {
          }
          frame 3, 6, 7 {
          }
        }
        n490 = And(x=w1066, y=w1064) -> (x .and. y?=w1065:bool)
        n491 = case shown="True" w1065 {
          tunnel: [w1072 _RT_Instrument_State."Running" ("InstrState")] -> w1070
          tunnel: w1067 -> [w1079 _]
          tunnel: w1061 -> [w1077 _]
          tunnel: w1064 -> [w1076 _]
          tunnel: w1063 -> [w1075 _]
          frame False {
            n492 = Select(t=_RT_Instrument_State."Shutting Down", s=w1077, f=w1079) -> (s? t:f=w1072:T3)
            n493 = Not Equal?(x=w1072, y=_RT_Instrument_State."Ready" ("t")) -> (x != y?=w1074:bool)
            n494 = case shown="True" w1074 {
              tunnel: w1072 -> [_ w1082]
              tunnel: w1076 -> [_ w1081]
              tunnel: w1075 -> [_ w1080]
              frame False {
              }
              frame True {
                n495 = Format Into String(format string="Instr State transitioned from Ready to %s; FPGA Running = %s; Run Mode = %d" ("Event"), w1082, w1081, w1080) -> (resulting string=w1083:string)  [unwired: 2 in, 1 out]
                n496 = call "_RT Event.vi"("Event"=w1083) -> ()  [unwired: 2 in, 5 out]
              }
            }
          }
          frame True {
            w1086 = T24 1 items=["Same", "Empty", "VacFail", "Cancel", "CheckGas", "EleFail", "Probe1Fail", "Probe2Fail", "HeaterFail", "DoorOpen", "CheckComm", "PressStart", "StartRP"] ("Line2Msg (same)")
            w1087 = T25 9 items=["Same", "Empty", "Connected", "Starting", "Stopping", "Action", "On", "Service", "Call", "Acquiring", "Source"] ("Line1Msg (same)")
            n497 = call "_FPGA Set LEDs.vi"("LED Command"=_LED_States."Solid B") -> ("error out"=w1088:errorcluster)  [unwired: 3 in, 3 out]
            n498 = call "_FPGA Set LCD Msg.vi"("error in"=w1088, "Line2Msg (same)"=w1086, "Line1Msg (same)"=w1087) -> ()  [unwired: 4 in, 3 out]
            n499 = call "_RT Event.vi"("Event"="A run has started") -> ()  [unwired: 2 in, 5 out]
          }
        }
      }
      frame "Source Standby" {
        n500 = global read "_RT Global.vi" "StartupMode"() -> (w1096:u8)
        n501 = case shown="2" w1096 {
          tunnel: [w1108 _RT_Instrument_State."Shutting Down" ("InstrState") _RT_Instrument_State."Starting Up" ("InstrState")] -> w1095
          tunnel: w1094 -> [w1105 _ _]
          tunnel: [w1100 w1110 w1112] -> w1093
          tunnel: w1092 -> [_ w1110 w1112]
          frame Default {
            w1099 = TRUE ("Waiting (F)")
            # "Allow system to shut down from this state"
            n502 = local read "Connected?"() -> (w1107:bool)
            n503 = call "_FPGA Read Key.vi"("CurStartupMode (0)"=u8 1) -> ("error out"=w1102:errorcluster, "Key Pressed"=w1101:bool, "Key Pressed 2"=w1100:bool)  [unwired: 3 in, 2 out]
            n504 = call "_FPGA System Polling.vi"("error in (no error)"=w1102, "Waiting (F)"=w1099, "Connected?"=w1107, "CurInstrState"=w1105, "High Vac Reached?"=w1099) -> ("Running"=w1106:bool, "Next InstrState"=w1104:T3)  [unwired: 2 out]
            n505 = local write "Running"(w1106) -> ()
            n506 = Select(t=_RT_Instrument_State."Shutting Down", s=w1101, f=w1104) -> (s? t:f=w1108:T3)
          }
          frame 2 {
            # "Received a shutdown command"
          }
          frame 0 {
            # "Received a startup command"
          }
        }
        n507 = local write "Fault"(TRUE ("Status LED")) -> ()
        n508 = local write "Ready"(FALSE ("Status LED")) -> ()
      }
      frame "Running" {
        n509 = local read "Connected?"() -> (w1117:bool)
        n510 = call "_FPGA System Polling.vi"("Connected?"=w1117, "CurInstrState"=w1118, "High Vac Reached?"=TRUE) -> ("Running"=w1119:bool, "Next InstrState"=w1120:T3)  [unwired: 2 in, 2 out]
        n511 = local write "Running"(w1119) -> ()
        n512 = case shown="True" w1119 {
          tunnel: [_RT_Instrument_State."Ready" ("InstrState") w1135] -> w1121
          tunnel: w1120 -> [_ w1135]
          tunnel: w1118 -> [_ w1137]
          frame False {
            w1122 = T24 1 items=["Same", "Empty", "VacFail", "Cancel", "CheckGas", "EleFail", "Probe1Fail", "Probe2Fail", "HeaterFail", "DoorOpen", "CheckComm", "PressStart", "StartRP"] ("Line2Msg (same)")
            w1123 = T25 6 items=["Same", "Empty", "Connected", "Starting", "Stopping", "Action", "On", "Service", "Call", "Acquiring", "Source"] ("Line1Msg (same)")
            n513 = call "_FPGA Set LEDs.vi"("LED Command"=_LED_States."Off BRP") -> ("error out"=w1124:errorcluster)  [unwired: 3 in, 3 out]
            n514 = local write "Fault"(FALSE ("Status LED")) -> ()
            n515 = call "_FPGA Set LEDs.vi"("error in (no error)"=w1124, "LED Command"=_LED_States."Solid P") -> ("error out"=w1126:errorcluster)  [unwired: 2 in, 3 out]
            n516 = local write "Ready"(TRUE ("Status LED")) -> ()
            n517 = call "_FPGA Set LCD Msg.vi"("error in"=w1126, "Line2Msg (same)"=w1122, "Line1Msg (same)"=w1123) -> ("error out"=w1127:errorcluster)  [unwired: 4 in, 2 out]
            n518 = call "_RT Event.vi"("Event"="A run ended normally, analyzer is ready") -> ()  [unwired: 2 in, 5 out]
            n519 = call "_FPGA Send LCD.vi"("error in (no error)"=w1127, "Command"=_RT_LED_Num."ReadKey" ("LED#")) -> ()  [unwired: 3 in, 4 out]
            n520 = global write "_RT Global.vi" "StartupMode"(u8 0 ("StartupMode")) -> ()
          }
          frame True {
            n521 = Not Equal?(x=w1137, y=w1135) -> (x != y?=w1136:bool)
            n522 = case shown="True" w1136 {
              tunnel: w1135 -> [_ w1142]
              frame False {
                n523 = call "_RT Event.vi"("Event"="Run in progress") -> ()  [unwired: 2 in, 5 out]
              }
              frame True {
                w1143 = u16 0 ("Address")
                # "End a Run"
                n524 = Format Into String(format string="A run unexpectedly ended as RT state changed from Running to %s.", w1142) -> (resulting string=w1140:string)  [unwired: 2 in, 1 out]
                n525 = call "_FPGA Set LEDs.vi"("LED Command"=_LED_States."Off B") -> ("error out"=w1139:errorcluster)  [unwired: 3 in, 3 out]
                n526 = call "_RT Event.vi"("Event"=w1140) -> ()  [unwired: 2 in, 5 out]
                n527 = call "_FPGA Write Data.vi"("error in"=w1139, "Data"=w1143, "Address"=w1143) -> ()  [unwired: 3 in, 3 out]
              }
            }
          }
        }
      }
      frame "Lost Communication" {
        # "Allow system to shutdown from this state"
        n528 = local read "Connected?"() -> (w1156:bool)
        n529 = call "_FPGA Read Key.vi"("CurStartupMode (0)"=u8 1) -> ("error out"=w1149:errorcluster, "Key Pressed"=w1148:bool, "Key Pressed 2"=w1147:bool)  [unwired: 3 in, 2 out]
        n530 = call "_FPGA System Polling.vi"("error in (no error)"=w1149, "Connected?"=w1156, "CurInstrState"=w1155, "High Vac Reached?"=TRUE) -> ("Running"=w1154:bool, "Next InstrState"=w1153:T3)  [unwired: 1 in, 2 out]
        n531 = local write "Running"(w1154) -> ()
        n532 = Select(t=_RT_Instrument_State."Shutting Down", s=w1148, f=w1153) -> (s? t:f=w1152:T3)
      }
      frame "Shutting Down" {
        # "button pressed"
        n533 = global read "_RT Global.vi" "StartupMode"() -> (w1157:u8)
        n534 = Equal?(x=w1157, y=u8 2) -> (x = y?=w1161:bool)
        n535 = Or(x=w1161, y=w1163) -> (x .or. y?=w1160:bool)
        n536 = case shown="True" w1160 {
          tunnel: ["Going to Roughing Pump Ready" ("Event") "Stopping Analyzer" ("Event")] -> w1159
          frame False {
          }
          frame True {
            n537 = global write "_RT Global.vi" "StartupMode"(u8 2 ("StartupMode")) -> ()
          }
        }
        n538 = Greater Than 0?(x=w1157) -> (x > 0?=w1169:bool)
        n539 = local read "Fault"() -> (w1172:bool)
        n540 = Or(x=w1172, y=w1169) -> (x .or. y?=w1171:bool)
        n541 = call "_RT Event.vi"("Event"=w1159) -> ("error out"=w1167:errorcluster)  [unwired: 2 in, 4 out]
        n542 = call "_Update Shutting Down.vi"("error in (no error)"=w1167, "Fault"=w1171) -> ("error Out"=w1165:errorcluster, "InstrState"=w1168:T3)  [unwired: 1 in, 3 out]
        n543 = local write "Ready"(FALSE ("Status LED")) -> ()
        n544 = call "_FPGA Send LCD.vi"("error in (no error)"=w1165, "Command"=_RT_LED_Num."ReadKey" ("LED#")) -> ()  [unwired: 2 in, 5 out]
      }
      frame "Fault" {
        # "Level 1 failure found and perform a total shutdown"
        n545 = stacked-sequence {
          frame #0 {
            n546 = local write "Ready"(FALSE ("Status LED")) -> ()
            n547 = call "_FPGA Set LEDs.vi"("LED Command"=_LED_States."Solid R") -> ()  [unwired: 3 in, 4 out]
            n548 = local write "Fault"(TRUE ("Status LED")) -> ()
            n549 = Wait (ms)(milliseconds to wait=u32 1800) -> ()  [unwired: 1 out]
          }
          frame #1 {
            n550 = call "_FPGA Send LCD.vi"("Command"=_RT_LED_Num."ReadKey" ("LED#")) -> ()  [unwired: 4 in, 4 out]
            n551 = global write "_RT Global.vi" "StartupMode"(u8 2 ("StartupMode")) -> ()
          }
        }
      }
    }
    n552 = global write "_RT Global.vi" "InstrState"(w812) -> ()
    n553 = Wait (ms)(milliseconds to wait=u32 280) -> ()  [unwired: 1 out]
    "InstrState" <- w812
  }
  n554 = while {
    shift-right: [w1185] -> _
    shift-left: w2 -> [w1194]
    tunnel: w1 -> [_]
    stop <- w1190 continue-if-true
    # "Laybold Pump HeartBeat - only send when not communicating with pump"
    n555 = global read "_RT Global.vi" "Leybold Pump ON"() -> (w1188:bool)
    n556 = Tick Count (ms)() -> (millisecond timer value=w1189:u32)
    n557 = global read "_RT Global.vi" "UseLeybold"() -> (w1190:bool)
    n558 = Subtract(x=w1189, y=w1194) -> (x-y=w1193:u32)
    n559 = Greater Or Equal?(x=w1193, y=u32 10000) -> (x >= y?=w1187:bool)
    n560 = Compound Arithmetic op=AND(w1190, w1188, w1187) -> (w1191:bool)
    n561 = case shown="True" w1191 {
      tunnel: w1194 -> [w1197 _]
      tunnel: [w1197 w1202] -> w1186
      tunnel: w1189 -> [_ w1202]
      frame False {
      }
      frame True {
        n562 = call "_FPGA Turbo Control.vi"("Command"=_Pump_Parameter."Read Actual Rotation Speed in Hz") -> ("Speed"=→"Speed":i32, "Error Code"=w1199:string)  [unwired: 3 in, 4 out]
        n563 = Empty String/Path?(string/path=w1199) -> (empty?=w1200:bool)
        n564 = case shown="False" w1200 {
          tunnel: w1199 -> [w1203 _]
          frame False {
            n565 = call "_RT Event.vi"("Event"=w1203) -> ()  [unwired: 2 in, 5 out]
          }
          frame True {
          }
        }
      }
    }
    n566 = flat-sequence {
      tunnel: w1186 -> [w1196]
      tunnel: [w1196] -> w1185
      frame #0 {
        n567 = Wait Until Next ms Multiple(millisecond multiple=u32 1000) -> ()  [unwired: 1 out]
      }
    }
  }
